vi "Convert_ERDs_JL.vi"(0 "New Header?":bool, 2 "ERD Name":string[](array[string]), 5 "ERD_Data_Bundled_Out":T1, 7 "Array":T11[](array[typedef]) {"ERD Number" format="%.0x"}, 11 "Error In":errorcluster) -> (6 "All_ERD_Data_Bundled_Brass":T1, 15 "Error Out":errorcluster)   [LabVIEW 2023]
doc: "This VI parses the data from ERDs in correct format, units, etc. It handles all hex to dec conversions, hex to enum, and hex to boolean conversions.\n\nIf Raw Data from ERD is blank string, then it will output values from shift register."
uses:
  Common/LabVIEW GEA2 Toolkit/GEA3/type defs/ERD Read Data Out.ctl
  type defs/All_Bundled_Data_JL.ctl
  Common/type defs/Version.ctl
  type defs/ERD_Always_Show_JL.ctl
  Common/type defs/CSV_File_String_Arrays.ctl
  Common/type defs/Fault Table Array.ctl
  Common/type defs/Fault_Table_Info.ctl
  type defs/Heat Control.ctl
  type defs/ERD_Commercial_Laundry.ctl
  Common/type defs/BootloaderVersion.ctl
  type defs/ERD_RJ45.ctl
panel:
  out "Numeric":i32
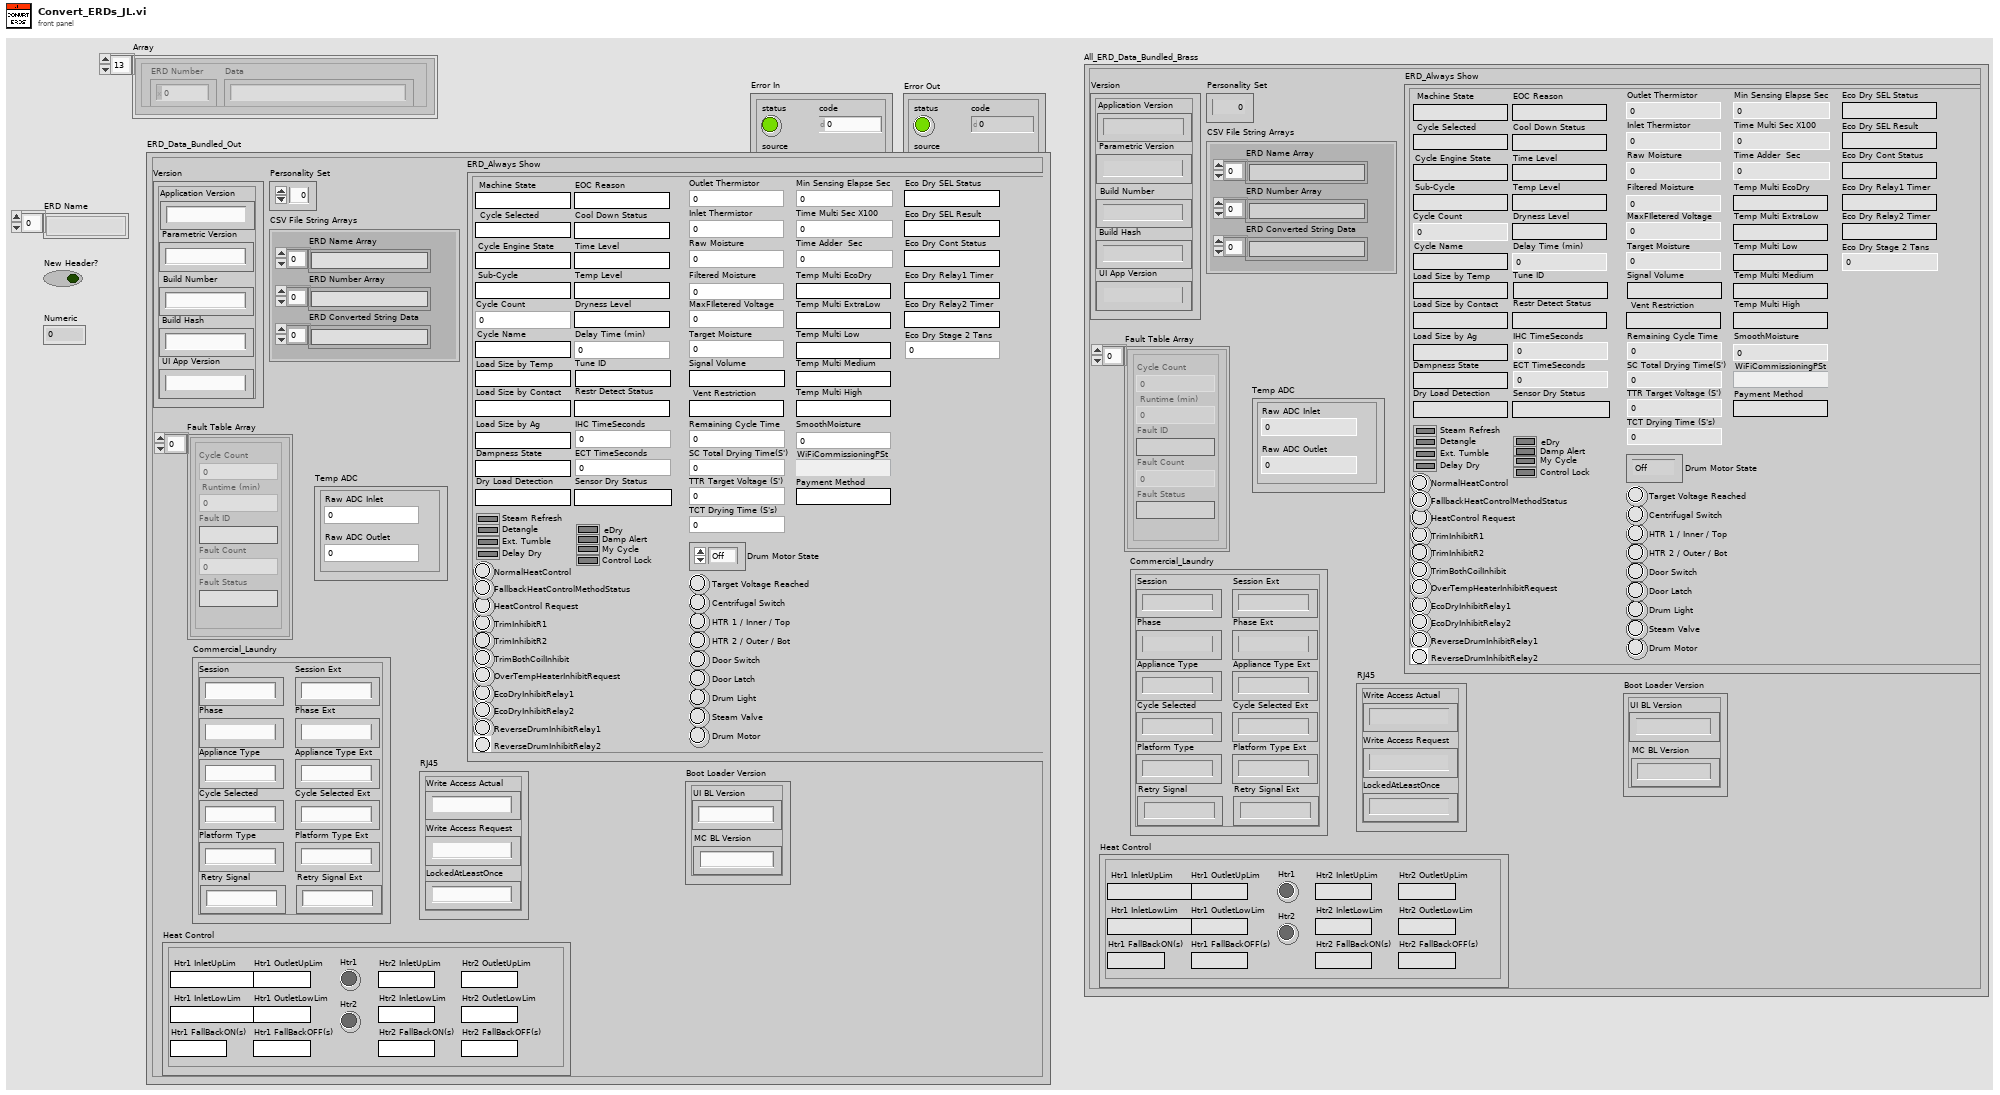
[diagram p1: front panel]
types:
  T1 = typedef "All_Bundled_Data_JL.ctl" = cluster{"Version":T2, "ERD_Always Show":T3, "Personality Set":u8, "CSV File String Arrays":T4, "Fault Table Array ":T5, "Heat Control":T7, "Temp ADC":cluster{"Raw ADC Outlet":u16, "Raw ADC Inlet":u16}, "Commercial_Laundry":T8, "Boot Loader Version":T9, "RJ45":T10}
  T2 = typedef "Version.ctl" = cluster{"Build Number":string, "Build Hash ":string, "Application Version":string, "Parametric Version":string, "UI App Version":string}
  T3 = typedef "ERD_Always_Show_JL.ctl" = cluster{"Inlet Thermistor":u16, "Machine State":string, "Filtered Moisture":u16, "Cycle Selected":string, "HTR 1 / Inner / Top":bool, "HTR 2 / Outer / Bot":bool, "Door Switch":bool, "Drum Light":bool, "Cycle Engine State":string, "Centrifugal Switch":bool, "Drum Motor":bool, "Cycle Count":u32, "Ext. Tumble":bool, "eDry":bool, "Temp Level":string, "Dryness Level":string, "Time Level":string, "Delay Time (min)":u16, "Steam Refresh":bool, "Damp Alert":bool, "Sub-Cycle":string, "Outlet Thermistor":u16, "Target Moisture":u16, "Remaining Cycle Time":u32, "Raw Moisture":u16, "Cycle Name":string, "My Cycle":bool, "Delay Dry":bool, "Detangle":bool, "Control Lock":bool, "Steam Valve":bool, "Door Latch":bool, "Signal Volume":string, "Tune ID":string, "Restr Detect Status":string, "Vent Restriction":string, "Load Size by Contact":string, "Load Size by Temp":string, "EOC Reason":string, "Sensor Dry Status":string, "Dampness State":string, "Target Voltage Reached":bool, "TrimInhibitR1":bool, "TrimInhibitR2":bool, "TrimBothCoilInhibit":bool, "NormalHeatControl":bool, "HeatControl Request":bool, "Cool Down Status":string, "EcoDryInhibitRelay1":bool, "EcoDryInhibitRelay2":bool, "ReverseDrumInhibitRelay1":bool, "ReverseDrumInhibitRelay2":bool, "OverTempHeaterInhibitRequest":bool, "FallbackHeatControlMethodStatus":bool, "IHC TimeSeconds":u32, "ECT TimeSeconds ":u32, "SC Total Drying Time(S')":u32, "TTR Target Voltage (S')":u32, "TCT Drying Time (S's)":u32, "Drum Motor State":enum16{"Off", "Cw", "Ccw", "Max"}, "Load Size by Ag":string, "MaxFIletered Voltage":u16, "Dry Load Detection":string, "Min Sensing Elapse Sec":u32, "Time Multi Sec X100":u32, "Time Adder  Sec":u32, "Temp Multi EcoDry":string, "Temp Multi ExtraLow":string, "Temp Multi Low ":string, "Temp Multi Medium":string, "Temp Multi High":string, "SmoothMoisture":u16, "Eco Dry SEL Status":string, "Eco Dry SEL Result":string, "Eco Dry Cont Status":string, "Eco Dry Relay1 Timer":string, "Eco Dry Relay2 Timer ":string, "Eco Dry Stage 2 Tans ":u32, "WiFiCommissioningPSt":string, "Payment Method":string}
  T4 = typedef "CSV_File_String_Arrays.ctl" = cluster{"ERD Number Array":string[], "ERD Name Array":string[], "ERD Converted String Data":string[]}
  T5 = typedef "Fault Table Array.ctl" = T6[]
  T6 = typedef "Fault_Table_Info.ctl" = cluster{"Cycle Count":u32, " Runtime (min) ":u32, "Fault Status":string, "Fault ID":string, "Fault Count":u16}
  T7 = typedef "Heat Control.ctl" = cluster{"Htr1 InletLowLim":string, "Htr1 InletUpLim":string, "Htr1 OutletLowLim":string, "Htr1 OutletUpLim":string, "Htr1 FallBackON(s)":string, "Htr1 FallBackOFF(s)":string, "Htr1":bool, "Htr2 InletLowLim":string, "Htr2 InletUpLim":string, "Htr2 OutletLowLim":string, "Htr2 OutletUpLim":string, "Htr2 FallBackON(s)":string, "Htr2 FallBackOFF(s)":string, "Htr2":bool}
  T8 = typedef "ERD_Commercial_Laundry.ctl" = cluster{"Session":string, "Phase":string, "Appliance Type":string, "Cycle Selected":string, "Platform Type":string, "Retry Signal":string, "Session Ext":string, "Phase Ext":string, "Appliance Type Ext":string, "Cycle Selected Ext":string, "Platform Type Ext":string, "Retry Signal Ext":string}
  T9 = typedef "BootloaderVersion.ctl" = cluster{"UI BL Version":string, "MC BL Version":string}
  T10 = typedef "ERD_RJ45.ctl" = cluster{"Write Access Actual":string, "Write Access Request":string, "LockedAtLeastOnce":string}
  T11 = typedef "ERD Read Data Out.ctl" = cluster{"ERD Number":u16, "Data":string}
  T12 = cluster{"Raw ADC Outlet":u16, "Raw ADC Inlet":u16}
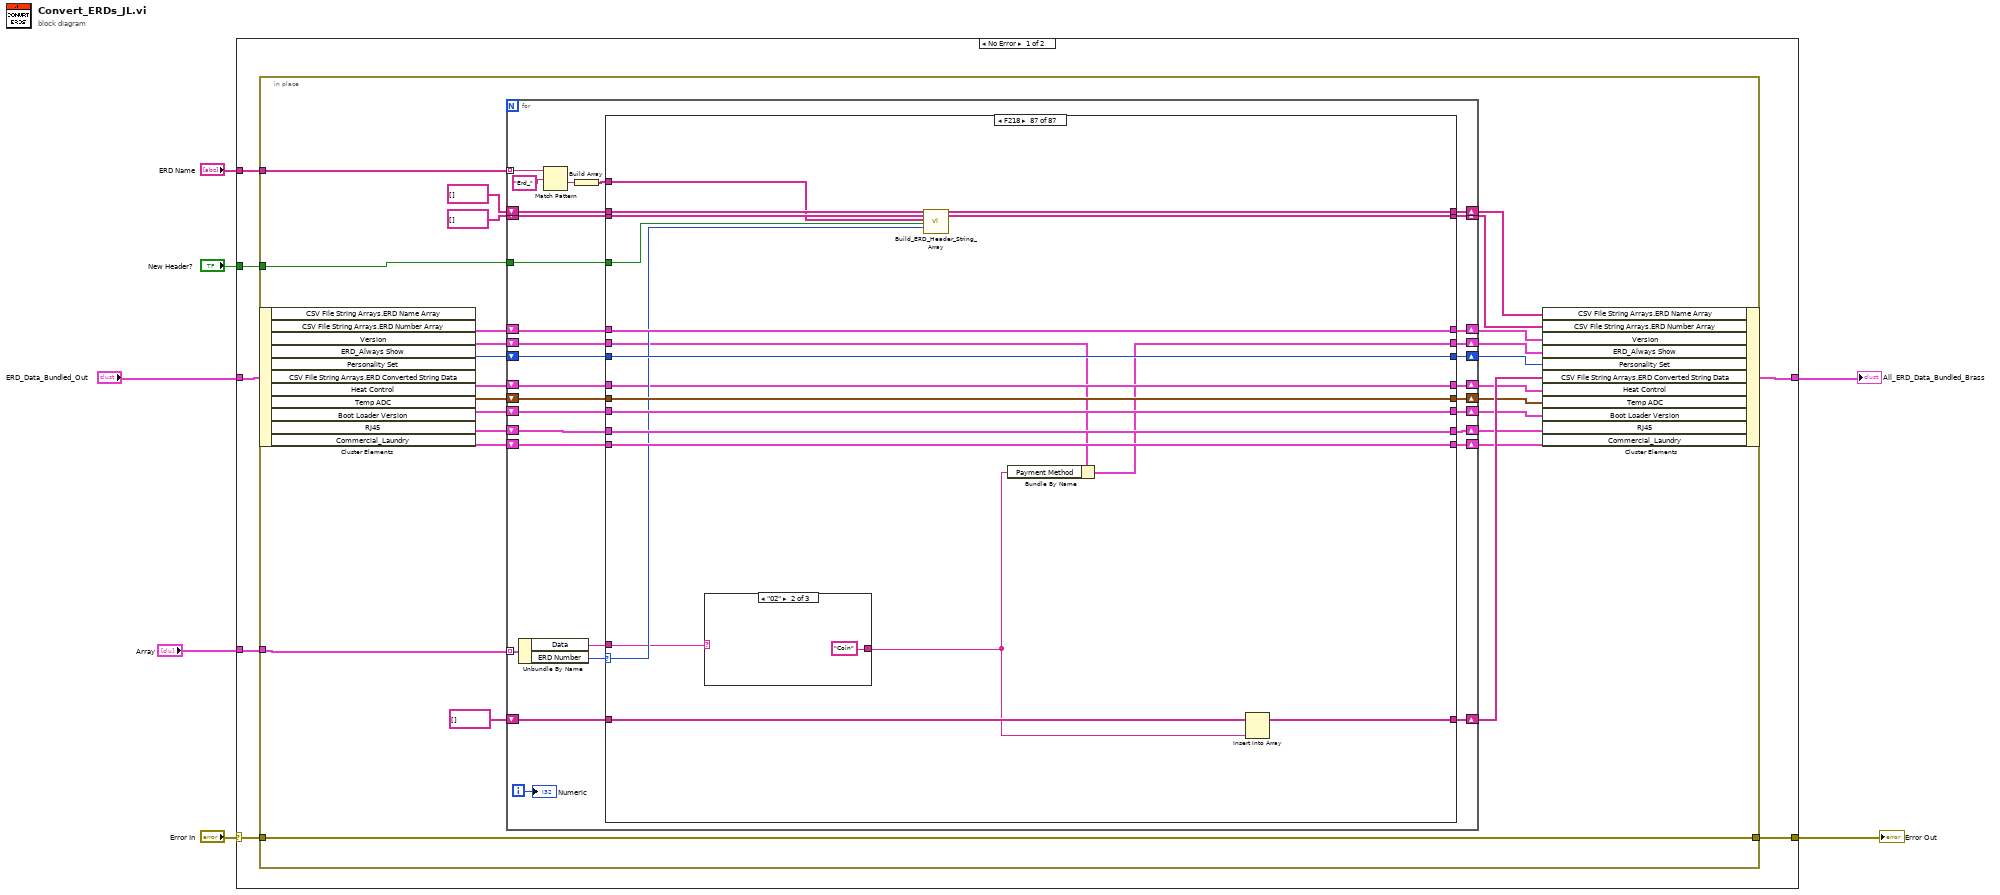
[diagram p0: block diagram]
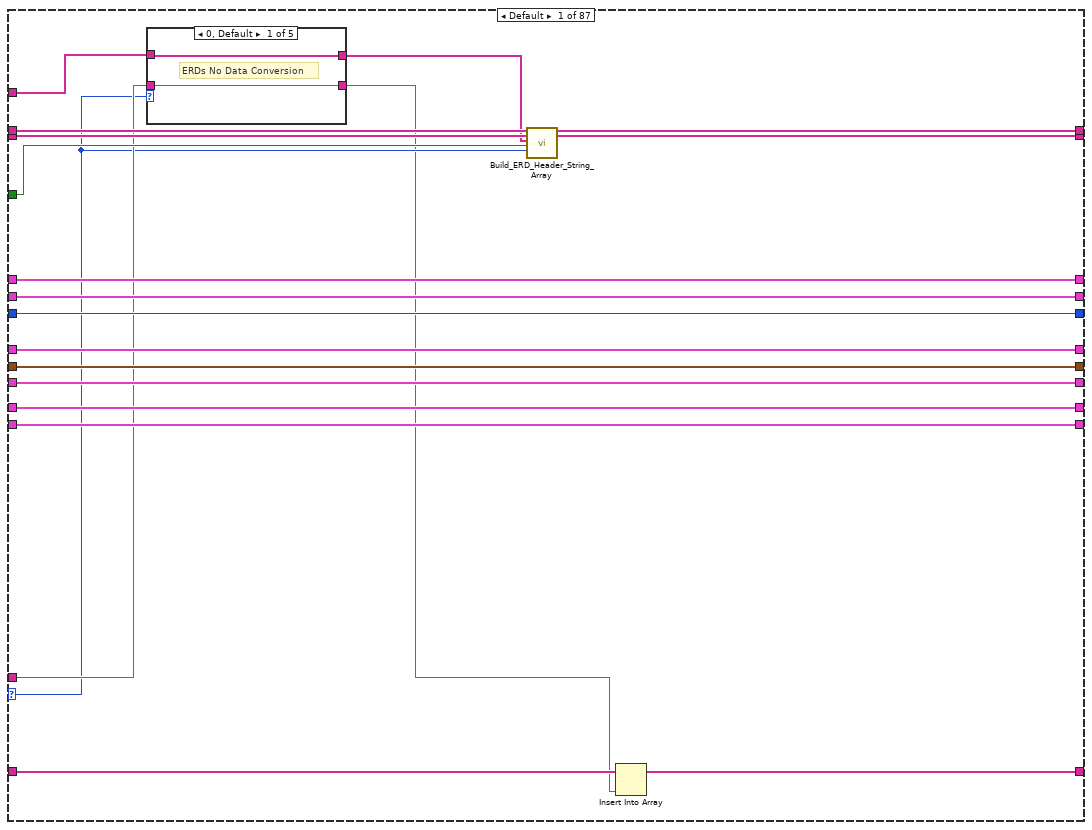
[diagram p2: hidden frame]
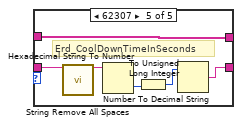
[diagram p6: hidden frame]
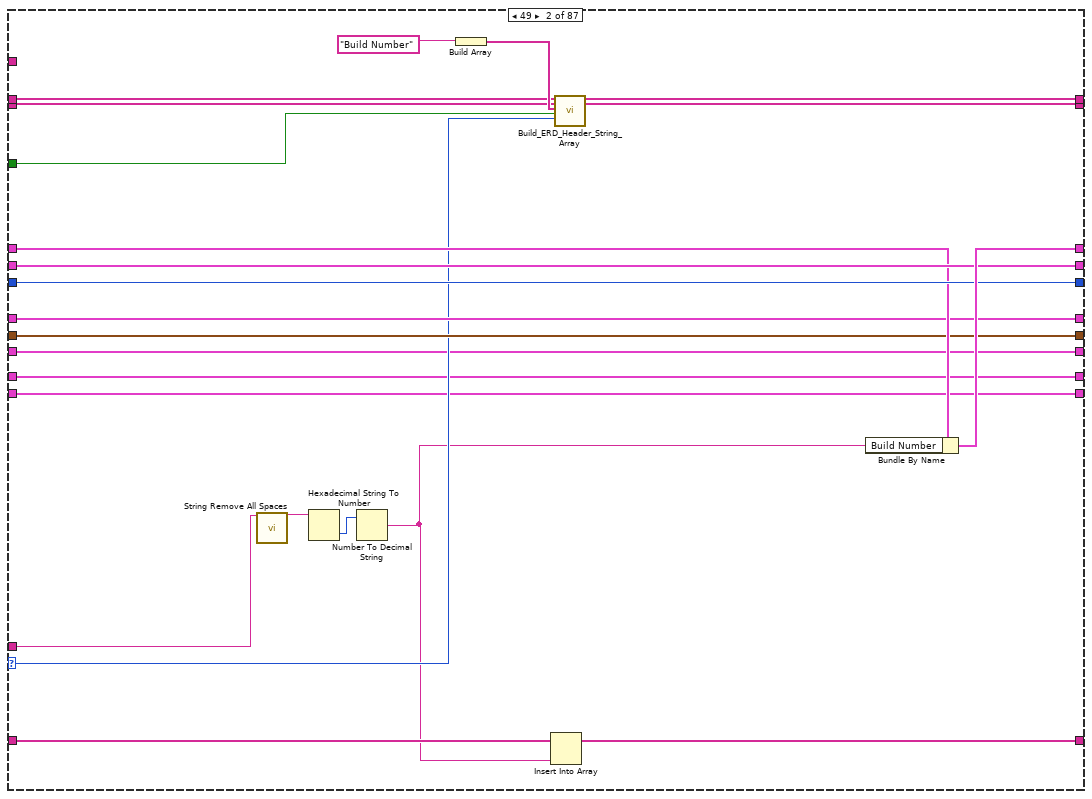
[diagram p7: hidden frame]
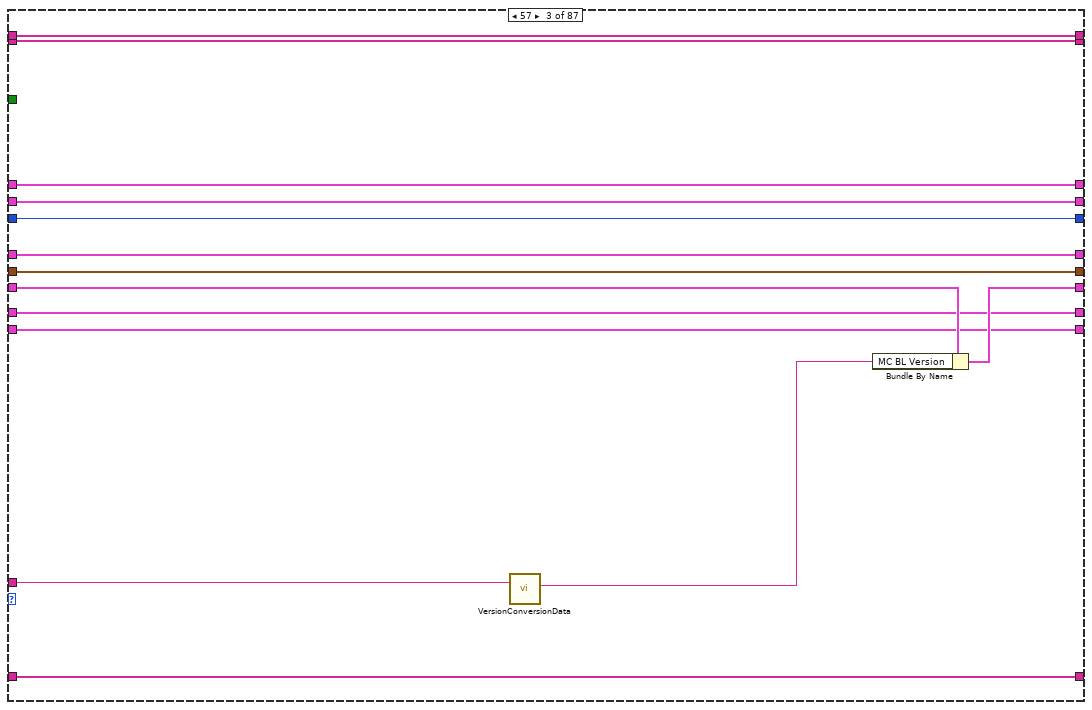
[diagram p8: hidden frame]
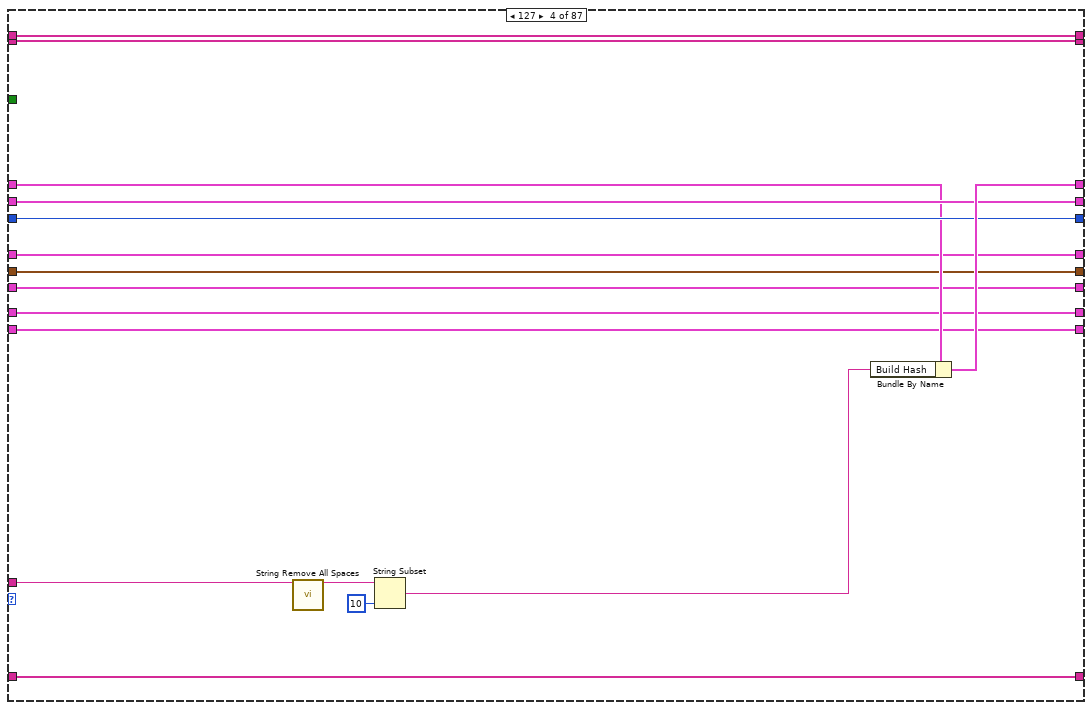
[diagram p9: hidden frame]
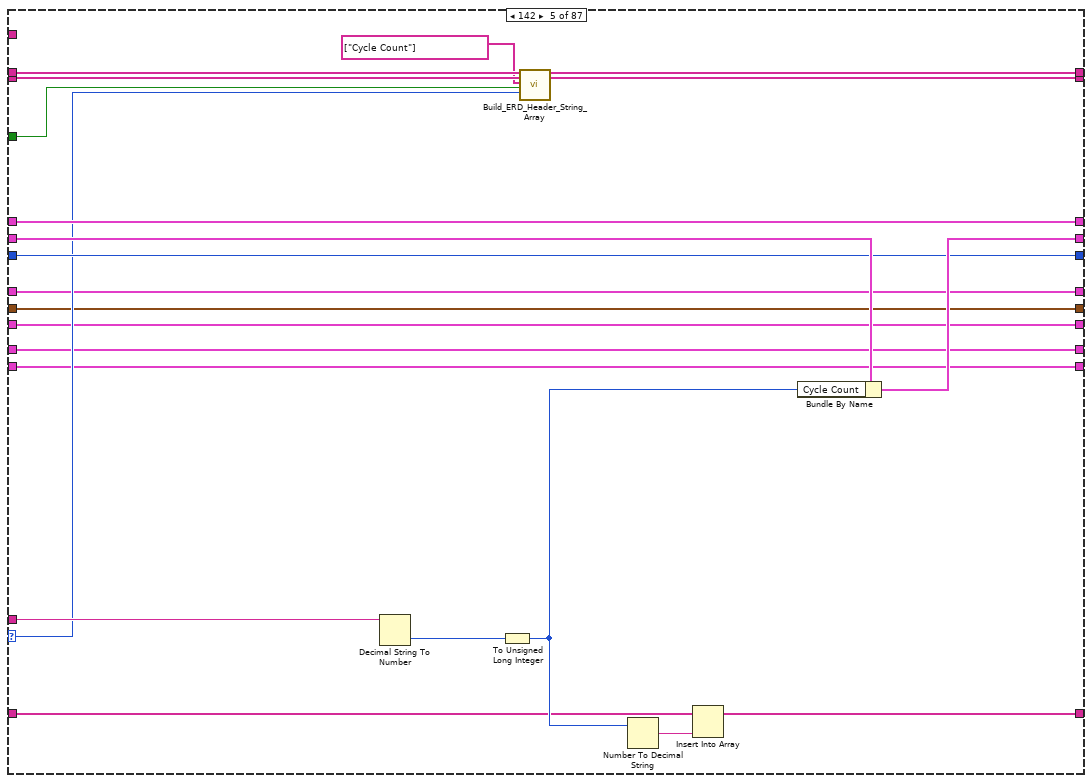
[diagram p10: hidden frame]
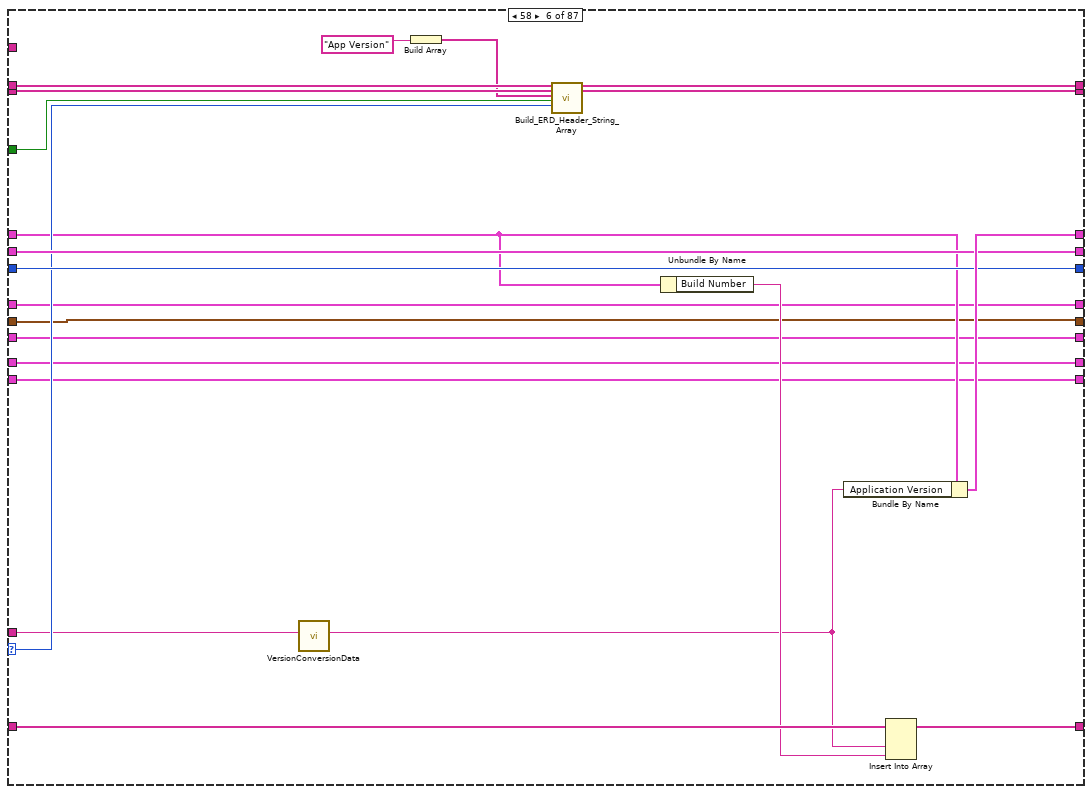
[diagram p11: hidden frame]
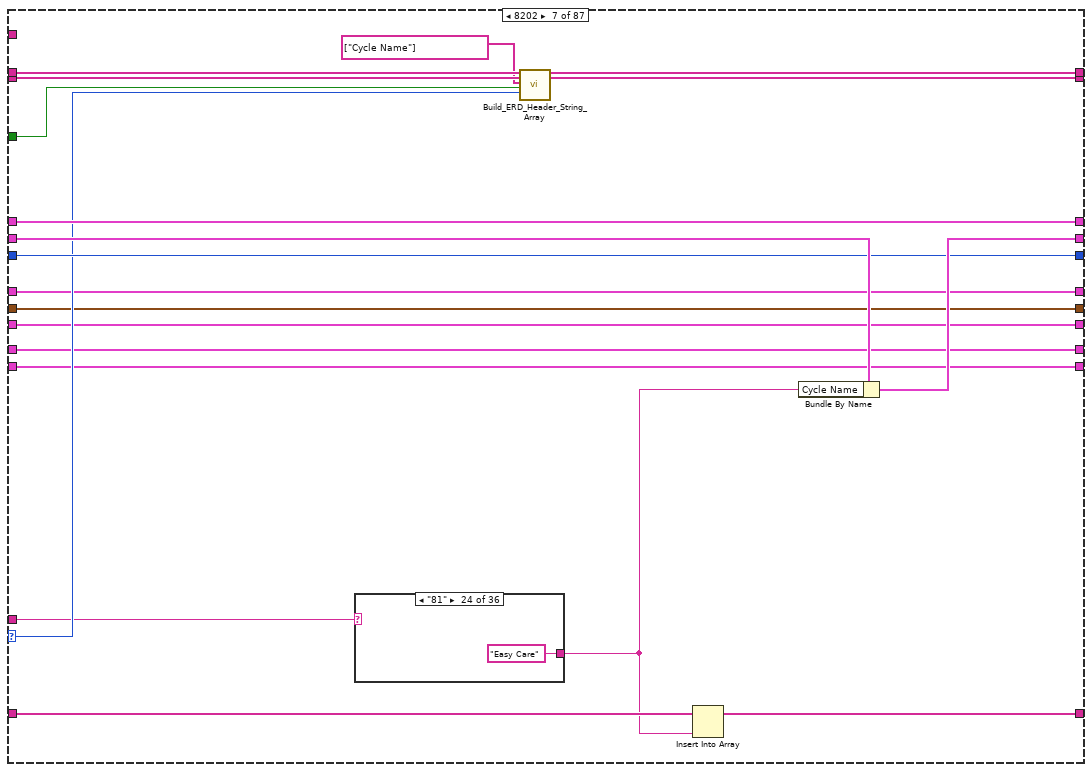
[diagram p12: hidden frame]
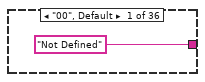
[diagram p13: hidden frame]
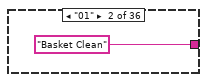
[diagram p14: hidden frame]
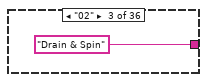
[diagram p15: hidden frame]
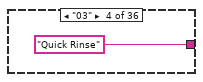
[diagram p16: hidden frame]
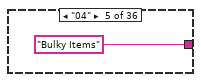
[diagram p17: hidden frame]
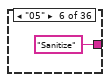
[diagram p18: hidden frame]
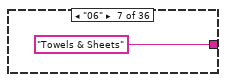
[diagram p19: hidden frame]
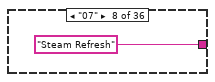
[diagram p20: hidden frame]
diagram:
  n1 = case shown="No Error" "Error In" {
    selector: "Error In" -> [w11 w2491]
    tunnel: "Array" -> [w14 _]
    tunnel: [w12 w2490] -> w5
    tunnel: "ERD_Data_Bundled_Out" -> [w13 w2489]
    tunnel: [w10 w2489] -> w4
    tunnel: "New Header?" -> [w9 _]
    tunnel: "ERD Name" -> [w8 _]
    frame No Error {
      n2 = in-place {
        in-place-border: w14 -> [w16]
        in-place-border: [w15] -> w12
        in-place-border: w11 -> [w15]
        in-place-border: w9 -> [w33]
        in-place-border: w8 -> [w21]
        n3 = in-place-cluster #1(w13) -> ("Version"=w39:T2, "ERD_Always Show"=w40:T3, "Personality Set"=w36:u8, "Heat Control"=w22:T7, "Temp ADC"=w25:T12, "Boot Loader Version"=w24:T9, "RJ45"=w19:T10, "Commercial_Laundry"=w17:T8)  [unwired: 3 out]
        n4 = for {
          shift-right: [w70] -> w37
          shift-left: w40 -> [w69]
          shift-right: [w67] -> w38
          shift-left: w39 -> [w68]
          shift-right: [w64] -> w35
          shift-left: w36 -> [w65]
          shift-right: [w62] -> w28
          shift-left: string[] [] ("ERD String Data") -> [w63]
          tunnel: w33 -> [w61]
          shift-right: [w57] -> w29
          shift-left: string[] [] ("ERD String Data") -> [w60]
          shift-right: [w58] -> w30
          shift-left: string[] [] ("ERD String Data") -> [w59]
          shift-right: [w50] -> w27
          shift-left: w22 -> [w56]
          shift-right: [w55] -> w26
          shift-left: w25 -> [w54]
          shift-right: [w51] -> w23
          shift-left: w24 -> [w52]
          tunnel: w21 -> [w49] mode=indexing
          shift-right: [w45] -> w20
          shift-left: w19 -> [w44]
          shift-right: [w43] -> w18
          shift-left: w17 -> [w42]
          tunnel: w16 -> [w41] mode=indexing
          i -> [w53]
          n5 = Unbundle By Name(w41) -> ("Data"=w71:string, "ERD Number"=w66:u16)
          n6 = Match Pattern(string=w49, regular expression="Erd_") -> (after substring=w46:string)  [unwired: 1 in, 3 out]
          n7 = Build Array(w46) -> (w47:string[])
          n8 = case shown="F218" w66 {
            selector: w66 -> [w73 w117 _ _ w169 w194 w212 w271 w296 w349 w380 w403 w431 w453 w498 w521 w544 w568 w587 w617 w649 w671 w694 w717 w740 w763 w787 w814 w836 w850 w877 w914 w933 w953 w982 w1005 w1036 w1063 w1086 w1111 w1135 w1158 w1181 w1203 w1226 w1272 w1290 w1313 w1336 w1359 w1382 w1405 w1428 w1451 w1471 w1499 w1554 w1612 w1642 w1673 w1693 w1722 w1747 w1770 w1793 w1816 w1842 w1872 w1897 w1920 w1937 w1965 w1988 w2011 w2037 w2061 w2081 w2102 w2143 w2170 w2188 w2212 w2239 w2266 w2313 w2406 w2478]
            tunnel: w71 -> [w74 w109 w130 w152 w180 w182 w209 w263 w289 w343 w393 w416 w427 w449 w468 w515 w538 w563 w595 w616 w648 w667 w691 w714 w737 w760 w782 w808 w828 w852 w883 w909 w930 w966 w981 w1016 w1046 w1077 w1100 w1121 w1149 w1172 w1195 w1216 w1239 w1267 w1301 w1324 w1347 w1370 w1393 w1416 w1439 w1462 w1485 w1492 w1564 w1622 w1652 w1684 w1704 w1732 w1758 w1781 w1804 w1827 w1853 w1865 w1889 w1912 w1947 w1964 w1987 w2010 w2048 w2053 w2092 w2112 w2141 w2167 w2182 w2205 w2233 w2260 w2282 w2375 w2469]
            tunnel: [w91 w127 w142 w157 w178 w201 w221 w279 w293 w358 w392 w415 w440 w462 w507 w530 w553 w576 w598 w629 w661 w685 w708 w731 w754 w777 w783 w804 w827 w859 w880 w907 w947 w965 w993 w1017 w1045 w1075 w1098 w1120 w1147 w1170 w1193 w1217 w1240 w1268 w1299 w1322 w1345 w1368 w1391 w1414 w1437 w1460 w1483 w1507 w1566 w1621 w1651 w1682 w1705 w1733 w1759 w1782 w1805 w1828 w1854 w1881 w1892 w1915 w1946 w1977 w2000 w2023 w2046 w2070 w2090 w2110 w2137 w2168 w2198 w2221 w2248 w2275 w2322 w2415 w2470] -> w70
            tunnel: w69 -> [w91 w127 w142 w157 w179 w201 w222 w279 w294 w359 w394 w417 w441 w463 w508 w531 w554 w577 w597 w630 w662 w682 w705 w728 w751 w774 w784 w805 w831 w858 w881 w908 w944 w967 w994 w1018 w1047 w1076 w1099 w1122 w1148 w1171 w1194 w1218 w1241 w1268 w1300 w1323 w1346 w1369 w1392 w1415 w1438 w1461 w1484 w1508 w1565 w1623 w1653 w1683 w1706 w1734 w1760 w1783 w1806 w1829 w1855 w1882 w1892 w1915 w1948 w1978 w2001 w2024 w2047 w2071 w2091 w2111 w2138 w2169 w2198 w2221 w2248 w2275 w2322 w2415 w2471]
            tunnel: w68 -> [w90 w125 w133 w153 w177 w193 w220 w278 w295 w357 w391 w414 w439 w461 w506 w529 w552 w575 w594 w628 w660 w684 w707 w730 w753 w776 w797 w806 w843 w870 w897 w924 w946 w964 w992 w1015 w1044 w1074 w1097 w1119 w1146 w1169 w1192 w1215 w1238 w1280 w1298 w1321 w1344 w1367 w1390 w1413 w1436 w1459 w1482 w1506 w1563 w1620 w1650 w1681 w1703 w1731 w1757 w1780 w1803 w1826 w1852 w1880 w1905 w1928 w1945 w1976 w1999 w2022 w2045 w2069 w2089 w2109 w2153 w2180 w2200 w2204 w2232 w2259 w2308 w2401 w2485]
            tunnel: [w90 w128 w133 w158 w177 w202 w220 w278 w295 w357 w391 w414 w439 w461 w506 w529 w552 w575 w594 w628 w660 w684 w707 w730 w753 w776 w797 w806 w843 w870 w897 w924 w946 w964 w992 w1015 w1044 w1074 w1097 w1119 w1146 w1169 w1192 w1215 w1238 w1280 w1298 w1321 w1344 w1367 w1390 w1413 w1436 w1459 w1482 w1506 w1563 w1620 w1650 w1681 w1703 w1731 w1757 w1780 w1803 w1826 w1852 w1880 w1905 w1928 w1945 w1976 w1999 w2022 w2045 w2069 w2089 w2109 w2153 w2180 w2199 w2204 w2232 w2259 w2308 w2401 w2485] -> w67
            tunnel: w65 -> [w89 w126 w141 w156 w176 w200 w219 _ w303 w356 w390 w413 w438 w460 w505 w528 w551 w574 w593 w627 w659 w681 w704 w727 w750 w773 w796 w821 w842 w869 w896 w923 w943 w963 w991 w1014 w1043 w1073 w1096 w1118 w1145 w1168 w1191 w1214 w1237 w1279 w1297 w1320 w1343 w1366 w1389 w1412 w1435 w1458 w1481 w1505 w1562 w1619 w1649 w1680 w1702 w1730 w1756 w1779 w1802 w1825 w1851 w1879 w1904 w1927 w1944 w1975 w1998 w2021 w2044 w2068 w2088 w2108 w2152 w2179 w2197 w2220 w2247 w2274 w2321 w2414 w2484]
            tunnel: [w89 w126 w141 w156 w176 w200 w219 w267 w303 w356 w390 w413 w438 w460 w505 w528 w551 w574 w593 w627 w659 w681 w704 w727 w750 w773 w796 w821 w842 w869 w896 w923 w943 w963 w991 w1014 w1043 w1073 w1096 w1118 w1145 w1168 w1191 w1214 w1237 w1279 w1297 w1320 w1343 w1366 w1389 w1412 w1435 w1458 w1481 w1505 w1562 w1619 w1649 w1680 w1702 w1730 w1756 w1779 w1802 w1825 w1851 w1879 w1904 w1927 w1944 w1975 w1998 w2021 w2044 w2068 w2088 w2108 w2152 w2179 w2197 w2220 w2247 w2274 w2321 w2414 w2484] -> w64
            tunnel: w63 -> [w85 w121 w138 w148 w174 w187 w217 w275 w300 w353 w384 w407 w435 w457 w502 w525 w548 w572 w591 w622 w653 w675 w698 w721 w744 w767 w791 w816 w834 w862 w887 w918 w937 w957 w987 w1011 w1040 w1067 w1090 w1115 w1139 w1162 w1185 w1208 w1231 w1276 w1294 w1317 w1340 w1363 w1386 w1409 w1432 w1455 w1475 w1503 w1558 w1616 w1646 w1677 w1699 w1728 w1753 w1776 w1799 w1822 w1848 w1876 w1901 w1924 w1941 w1969 w1992 w2015 w2041 w2065 w2085 w2106 w2148 w2174 w2192 w2216 w2243 w2270 w2317 w2410 w2474]
            tunnel: [w81 w120 w138 w148 w172 w196 w215 w273 w298 w351 w382 w405 w433 w455 w500 w523 w546 w570 w589 w620 w651 w673 w696 w719 w742 w765 w789 w812 w837 w865 w886 w916 w935 w955 w985 w1009 w1038 w1065 w1088 w1113 w1137 w1160 w1183 w1206 w1229 w1274 w1292 w1315 w1338 w1361 w1384 w1407 w1430 w1453 w1473 w1501 w1556 w1614 w1644 w1675 w1697 w1726 w1751 w1774 w1797 w1820 w1846 w1874 w1899 w1922 w1939 w1967 w1990 w2013 w2039 w2063 w2083 w2104 w2146 w2172 w2190 w2214 w2241 w2268 w2315 w2408 w2476] -> w62
            tunnel: w61 -> [w83 w115 _ _ w170 w195 w213 w272 w297 w350 w381 w404 w432 w454 w499 w522 w545 w569 w588 w619 w650 w672 w695 w718 w741 w764 w788 w815 w835 w861 w884 w915 w934 w954 w984 w1006 w1037 w1064 w1087 w1112 w1136 w1159 w1182 w1205 w1228 w1273 w1291 w1314 w1337 w1360 w1383 w1406 w1429 w1452 w1472 w1500 w1555 w1613 w1643 w1674 w1694 w1723 w1748 w1771 w1794 w1817 w1843 w1873 w1898 w1921 w1938 w1966 w1989 w2012 w2038 w2062 w2082 w2103 w2144 w2171 w2189 w2213 w2240 w2267 w2314 w2407 w2479]
            tunnel: w60 -> [w84 w119 w139 w154 w175 w188 w218 w276 w301 w354 w385 w408 w436 w458 w503 w526 w549 w573 w592 w623 w654 w676 w699 w722 w745 w768 w792 w817 w833 w863 w888 w919 w938 w958 w988 w1012 w1041 w1068 w1091 w1116 w1140 w1163 w1186 w1209 w1232 w1277 w1295 w1318 w1341 w1364 w1387 w1410 w1433 w1456 w1476 w1504 w1559 w1617 w1647 w1678 w1700 w1729 w1754 w1777 w1800 w1823 w1849 w1877 w1902 w1925 w1942 w1970 w1993 w2016 w2042 w2066 w2086 w2107 w2149 w2175 w2193 w2217 w2244 w2271 w2318 w2411 w2475]
            tunnel: w59 -> [w79 w113 w140 w155 w165 w199 w211 w269 w286 w346 w388 w411 w430 w452 w497 w520 w543 w567 w586 w625 w657 w679 w702 w725 w748 w771 w786 w810 w829 w856 w882 w911 w941 w962 w990 w1008 w1035 w1071 w1094 w1110 w1143 w1166 w1189 w1212 w1235 w1269 w1289 w1312 w1335 w1358 w1381 w1404 w1427 w1450 w1479 w1498 w1561 w1611 w1641 w1672 w1696 w1725 w1750 w1773 w1796 w1819 w1845 w1871 w1896 w1919 w1936 w1973 w1996 w2019 w2035 w2059 w2080 w2101 w2140 w2166 w2196 w2219 w2246 w2273 w2320 w2413 w2468]
            tunnel: [w80 w112 w140 w155 w164 w198 w210 w268 w285 w345 w387 w410 w429 w451 w496 w519 w542 w566 w585 w624 w656 w678 w701 w724 w747 w770 w785 w809 w830 w857 w878 w912 w940 w961 w989 w1007 w1034 w1070 w1093 w1109 w1142 w1165 w1188 w1211 w1234 w1271 w1288 w1311 w1334 w1357 w1380 w1403 w1426 w1449 w1478 w1497 w1560 w1610 w1640 w1671 w1695 w1724 w1749 w1772 w1795 w1818 w1844 w1870 w1895 w1918 w1935 w1972 w1995 w2018 w2034 w2058 w2079 w2100 w2135 w2165 w2195 w2218 w2245 w2272 w2319 w2412 w2467] -> w58
            tunnel: [w82 w118 w139 w154 w173 w197 w216 w274 w299 w352 w383 w406 w434 w456 w501 w524 w547 w571 w590 w621 w652 w674 w697 w720 w743 w766 w790 w813 w838 w864 w885 w917 w936 w956 w986 w1010 w1039 w1066 w1089 w1114 w1138 w1161 w1184 w1207 w1230 w1275 w1293 w1316 w1339 w1362 w1385 w1408 w1431 w1454 w1474 w1502 w1557 w1615 w1645 w1676 w1698 w1727 w1752 w1775 w1798 w1821 w1847 w1875 w1900 w1923 w1940 w1968 w1991 w2014 w2040 w2064 w2084 w2105 w2147 w2173 w2191 w2215 w2242 w2269 w2316 w2409 w2477] -> w57
            tunnel: w56 -> [w86 w124 w137 w147 w163 w191 w207 w266 w284 w339 w378 w401 w426 w448 w495 w517 w540 w564 w583 w614 w639 w669 w692 w715 w738 w761 w781 w811 w826 w855 w879 w913 w931 w952 w979 w1003 w1032 w1061 w1085 w1107 w1133 w1156 w1179 w1202 w1225 w1270 w1285 w1308 w1331 w1354 w1377 w1400 w1423 w1446 w1469 w1496 w1553 w1609 w1639 w1668 w1691 w1720 w1745 w1768 w1791 w1814 w1840 w1868 w1893 w1916 w1934 w1962 w1985 w2008 w2031 w2055 w2076 w2099 w2145 w2177 w2187 w2211 w2238 w2265 w2312 w2405 w2472]
            tunnel: [w86 w124 w137 w147 w163 w191 w207 w266 w284 w339 w378 w401 w426 w448 w495 w517 w540 w564 w583 w614 w639 w669 w692 w715 w738 w761 w781 w811 w826 w855 w879 w913 w931 w952 w979 w1003 w1032 w1061 w1085 w1107 w1133 w1156 w1179 w1202 w1225 w1264 w1285 w1308 w1331 w1354 w1377 w1400 w1423 w1446 w1469 w1496 w1553 w1609 w1639 w1668 w1691 w1720 w1745 w1768 w1791 w1814 w1840 w1868 w1893 w1916 w1934 w1962 w1985 w2008 w2031 w2055 w2076 w2099 w2145 w2177 w2187 w2211 w2238 w2265 w2312 w2405 w2472] -> w50
            tunnel: w54 -> [w88 w123 w136 w146 w162 w190 w206 w265 w283 w328 w377 w400 w425 w447 w494 w516 w539 w561 w582 w613 w638 w668 w689 w712 w735 w758 w795 w820 w841 w868 w895 w922 w928 w951 w978 w1002 w1031 w1060 w1084 w1106 w1132 w1155 w1178 w1201 w1224 w1261 w1284 w1307 w1330 w1353 w1376 w1399 w1422 w1445 w1468 w1495 w1552 w1607 w1637 w1667 w1690 w1719 w1744 w1767 w1790 w1813 w1839 w1867 w1891 w1914 w1932 w1961 w1984 w2007 w2030 w2054 w2075 w2098 w2151 w2178 w2186 w2210 w2237 w2264 w2311 w2404 w2483]
            tunnel: [w88 w123 w136 w146 w162 w190 w206 w265 w283 w328 w377 w400 w425 w447 w494 w516 w539 w561 w582 w613 w638 w668 w689 w712 w735 w758 w795 w820 w841 w868 w895 w922 w928 w951 w978 w1002 w1031 w1060 w1084 w1106 w1132 w1155 w1178 w1201 w1224 w1261 w1284 w1307 w1330 w1353 w1376 w1399 w1422 w1445 w1468 w1495 w1552 w1607 w1637 w1667 w1690 w1719 w1744 w1767 w1790 w1813 w1839 w1867 w1890 w1913 w1932 w1961 w1984 w2007 w2030 w2054 w2075 w2098 w2151 w2178 w2186 w2210 w2237 w2264 w2311 w2404 w2483] -> w55
            tunnel: w52 -> [w87 w114 w135 w145 w161 w189 w205 w264 w282 w327 w376 w399 w422 w444 w466 w511 w534 w558 w581 w612 w637 w665 w688 w711 w734 w757 w794 w819 w840 w867 w894 w921 w927 w950 w977 w1001 w1030 w1059 w1082 w1105 w1131 w1154 w1177 w1200 w1223 w1246 w1283 w1306 w1329 w1352 w1375 w1398 w1421 w1444 w1467 w1494 w1551 w1606 w1636 w1666 w1689 w1718 w1743 w1766 w1789 w1812 w1838 w1862 w1885 w1908 w1931 w1960 w1983 w2006 w2029 w2051 w2074 w2097 w2150 w2163 w2185 w2209 w2236 w2263 w2310 w2403 w2482]
            tunnel: [w87 w114 w134 w145 w161 w189 w205 w264 w282 w327 w376 w399 w422 w444 w466 w511 w534 w558 w581 w612 w637 w665 w688 w711 w734 w757 w794 w819 w840 w867 w894 w921 w927 w950 w977 w1001 w1030 w1059 w1082 w1105 w1131 w1154 w1177 w1200 w1223 w1246 w1283 w1306 w1329 w1352 w1375 w1398 w1421 w1444 w1467 w1494 w1551 w1606 w1636 w1666 w1689 w1718 w1743 w1766 w1789 w1812 w1838 w1862 w1885 w1908 w1931 w1960 w1983 w2006 w2029 w2051 w2074 w2097 w2150 w2163 w2185 w2209 w2236 w2263 w2310 w2403 w2482] -> w51
            tunnel: w47 -> [w77 _ _ _ _ _ _ w261 _ _ _ _ _ _ _ _ _ w557 w580 _ _ _ _ _ _ _ _ _ _ _ _ _ _ _ _ _ _ _ _ _ _ _ _ _ _ _ _ _ _ _ _ _ _ _ _ w1493 w1548 _ _ _ _ w1717 _ _ _ _ _ _ _ _ _ _ _ _ _ _ _ _ w2134 _ _ _ _ _ _ _ w2473]
            tunnel: [w76 w111 w132 w144 w160 w184 w204 w260 w281 w326 w375 w398 w421 w443 w465 w510 w533 w556 w579 w611 w636 w664 w687 w710 w733 w756 w780 w803 w825 w849 w876 w903 w926 w949 w976 w1000 w1029 w1058 w1081 w1104 w1130 w1153 w1176 w1199 w1222 w1245 w1282 w1305 w1328 w1351 w1374 w1397 w1420 w1443 w1466 w1489 w1547 w1605 w1635 w1665 w1688 w1716 w1742 w1765 w1788 w1811 w1837 w1861 w1884 w1907 w1930 w1959 w1982 w2005 w2028 w2050 w2073 w2096 w2133 w2162 w2184 w2202 w2230 w2257 w2306 w2399 w2481] -> w45
            tunnel: w44 -> [w76 w111 w132 w144 w160 w184 w204 w260 w281 w326 w375 w398 w421 w443 w465 w510 w533 w556 w579 w611 w636 w664 w687 w710 w733 w756 w780 w803 w825 w849 w876 w903 w926 w949 w976 w1000 w1029 w1058 w1081 w1104 w1130 w1153 w1176 w1199 w1222 w1245 w1282 w1305 w1328 w1351 w1374 w1397 w1420 w1443 w1466 w1489 w1547 w1605 w1635 w1665 w1688 w1716 w1742 w1765 w1788 w1811 w1837 w1861 w1884 w1907 w1930 w1959 w1982 w2005 w2028 w2050 w2073 w2096 w2133 w2162 w2184 w2203 w2231 w2258 w2306 w2399 w2481]
            tunnel: [w75 w110 w131 w143 w159 w183 w203 w259 w280 w325 w374 w397 w420 w442 w464 w509 w532 w555 w578 w610 w635 w663 w686 w709 w732 w755 w779 w802 w824 w848 w875 w902 w925 w948 w975 w999 w1028 w1057 w1080 w1103 w1129 w1152 w1175 w1198 w1221 w1244 w1281 w1304 w1327 w1350 w1373 w1396 w1419 w1442 w1465 w1488 w1546 w1604 w1634 w1664 w1687 w1715 w1741 w1764 w1787 w1810 w1836 w1860 w1883 w1906 w1929 w1958 w1981 w2004 w2027 w2049 w2072 w2095 w2132 w2161 w2183 w2208 w2235 w2262 w2281 w2374 w2480] -> w43
            tunnel: w42 -> [w75 w110 w131 w143 w159 w183 w203 w259 w280 w325 w374 w397 w420 w442 w464 w509 w532 w555 w578 w610 w635 w663 w686 w709 w732 w755 w779 w802 w824 w848 w875 w902 w925 w948 w975 w999 w1028 w1057 w1080 w1103 w1129 w1152 w1175 w1198 w1221 w1244 w1281 w1304 w1327 w1350 w1373 w1396 w1419 w1442 w1465 w1488 w1546 w1604 w1634 w1664 w1687 w1715 w1741 w1764 w1787 w1810 w1836 w1860 w1883 w1906 w1929 w1958 w1981 w2004 w2027 w2049 w2072 w2095 w2132 w2161 w2183 w2208 w2235 w2262 w2305 w2398 w2480]
            frame Default {
              n9 = case shown="0, Default" w73 {
                tunnel: [w92 w95 w97 w99 w105] -> w78
                tunnel: w77 -> [w92 w95 w97 w99 w105]
                tunnel: w74 -> [w93 w94 w96 w98 w102]
                tunnel: [w93 w94 w96 w98 w100] -> w72
                frame 0, Default {
                  # "ERDs No Data Conversion"
                }
                frame 65423 {
                  # "Consumer Error Mode"
                }
                frame 55 {
                  # "ServiceModeState"
                }
                frame 61811 {
                  # "WiFiCommissioningOption"
                }
                frame 62307 {
                  # "Erd_CoolDownTimeInSeconds"
                  n10 = call "String Remove All Spaces.vi"("Input String"=w102) -> ("Spaces Removed"=w103:string)  [unwired: 13 in, 1 out]
                  n11 = Hexadecimal String To Number(string=w103) -> (number=w104:u32)  [unwired: 2 in, 1 out]
                  n12 = To Unsigned Long Integer(number=w104) -> (unsigned 32bit integer=w101:u32)
                  n13 = Number To Decimal String(number=w101) -> (decimal integer string=w100:string)  [unwired: 1 in]
                }
              }
              n14 = call "Build_ERD_Header_String_Array.vi"("ERD Name Array In"=w84, "ERD Number Array In"=w85, "ERD Name List"=w78, "New Header?"=w83, "ERD Number"=w73) -> ("ERD Name Array Out"=w82:string[], "ERD Number Array Out"=w81:string[])  [unwired: 13 in]
              n15 = Insert Into Array(array=w79, new element=w72) -> (w80:string[])  [unwired: 1 in]
            }
            frame 49 {
              n16 = call "String Remove All Spaces.vi"("Input String"=w109) -> ("Spaces Removed"=w108:string)  [unwired: 13 in, 1 out]
              n17 = Hexadecimal String To Number(string=w108) -> (number=w106:u32)  [unwired: 2 in, 1 out]
              n18 = Number To Decimal String(number=w106) -> (decimal integer string=w107:string)  [unwired: 1 in]
              n19 = Build Array("Build Number") -> (w122:string[])
              n20 = Insert Into Array(array=w113, new element=w107) -> (w112:string[])  [unwired: 1 in]
              n21 = call "Build_ERD_Header_String_Array.vi"("ERD Name Array In"=w119, "ERD Number Array In"=w121, "ERD Name List"=w122, "New Header?"=w115, "ERD Number"=w117) -> ("ERD Name Array Out"=w118:string[], "ERD Number Array Out"=w120:string[])  [unwired: 13 in]
              n22 = Bundle By Name(cluster=w125, "Build Number"=w107) -> (w128:T2)
            }
            frame 57 {
              n23 = call "VersionConversionData.vi"("Version In"=w130) -> ("Version Out"=w129:string)  [unwired: 9 in, 1 out]
              n24 = Bundle By Name(cluster=w135, "MC BL Version"=w129) -> (w134:T9)
            }
            frame 127 {
              n25 = call "String Remove All Spaces.vi"("Input String"=w152) -> ("Spaces Removed"=w151:string)  [unwired: 13 in, 1 out]
              n26 = String Subset(string=w151, length (rest)=10 ("length (rest)")) -> (substring=w149:string)  [unwired: 1 in]
              n27 = Bundle By Name(cluster=w153, "Build Hash"=w149) -> (w158:T2)
            }
            frame 142 {
              n28 = Decimal String To Number(string=w180) -> (number=w167:i32)  [unwired: 2 in, 1 out]
              n29 = To Unsigned Long Integer(number=w167) -> (unsigned 32bit integer=w166:u32)
              n30 = call "Build_ERD_Header_String_Array.vi"("ERD Name Array In"=w175, "ERD Number Array In"=w174, "ERD Name List"=string[] ["Cycle Count"], "New Header?"=w170, "ERD Number"=w169) -> ("ERD Name Array Out"=w173:string[], "ERD Number Array Out"=w172:string[])  [unwired: 13 in]
              n31 = Number To Decimal String(number=w166) -> (decimal integer string=w168:string)  [unwired: 1 in]
              n32 = Insert Into Array(array=w165, new element=w168) -> (w164:string[])  [unwired: 1 in]
              n33 = Bundle By Name(cluster=w179, "Cycle Count"=w166) -> (w178:T3)
            }
            frame 58 {
              n34 = call "VersionConversionData.vi"("Version In"=w182) -> ("Version Out"=w181:string)  [unwired: 9 in, 1 out]
              n35 = Build Array("App Version" ("String")) -> (w185:string[])
              n36 = call "Build_ERD_Header_String_Array.vi"("ERD Name Array In"=w188, "ERD Number Array In"=w187, "ERD Name List"=w185, "New Header?"=w195, "ERD Number"=w194) -> ("ERD Name Array Out"=w197:string[], "ERD Number Array Out"=w196:string[])  [unwired: 13 in]
              n37 = Unbundle By Name(w193) -> ("Build Number"=w192:string)
              n38 = Bundle By Name(cluster=w193, "Application Version"=w181) -> (w202:T2)
              n39 = Insert Into Array(array=w199, new element #1=w181, new element #2=w192) -> (w198:string[])  [unwired: 1 in]
            }
            frame 8202 {
              n40 = case shown="\"81\"" w209 {
                tunnel: ["Not Defined" "Basket Clean" "Drain & Spin" "Quick Rinse" "Bulky Items" "Sanitize" "Towels & Sheets" "Steam Refresh" "Normal/Mixed" "Whites" "Dark Colors" "Jeans" "Hand Wash" "Delicates" "Speed Wash" "Heavy Duty" "Allergen" "Power Clean" "Rinse & Spin" "Single Item" "Colors" "Cold Wash" "Cottons" "Easy Care" "Active Wear" "Timed Dry" "Dewrinkle" "Air Fluff" "Steam Refresh" "Steam Dewrinkle" "Speed Dry" "Mixed" "Quick Dry" "Casuals" "Warm Up" "Energy Saver"] -> w208
                frame "00", Default {
                }
                frame "01" {
                }
                frame "02" {
                }
                frame "03" {
                }
                frame "04" {
                }
                frame "05" {
                }
                frame "06" {
                }
                frame "07" {
                }
                frame "08" {
                }
                frame "09" {
                }
                frame "0A" {
                }
                frame "0B" {
                }
                frame "0C" {
                }
                frame "0D" {
                }
                frame "0E" {
                }
                frame "0F" {
                }
                frame "10" {
                }
                frame "11" {
                }
                frame "12" {
                }
                frame "13" {
                }
                frame "14" {
                }
                frame "15" {
                }
                frame "80" {
                }
                frame "81" {
                }
                frame "82" {
                }
                frame "83" {
                }
                frame "84" {
                }
                frame "85" {
                }
                frame "86" {
                }
                frame "87" {
                }
                frame "88" {
                }
                frame "89" {
                }
                frame "8A" {
                }
                frame "8B" {
                }
                frame "8C" {
                }
                frame "8D" {
                }
              }
              n41 = call "Build_ERD_Header_String_Array.vi"("ERD Name Array In"=w218, "ERD Number Array In"=w217, "ERD Name List"=string[] ["Cycle Name"], "New Header?"=w213, "ERD Number"=w212) -> ("ERD Name Array Out"=w216:string[], "ERD Number Array Out"=w215:string[])  [unwired: 13 in]
              n42 = Insert Into Array(array=w211, new element=w208) -> (w210:string[])  [unwired: 1 in]
              n43 = Bundle By Name(cluster=w222, "Cycle Name"=w208) -> (w221:T3)
            }
            frame 65281 {
              n44 = call "String Remove All Spaces.vi"("Input String"=w263) -> ("Spaces Removed"=w262:string)  [unwired: 13 in, 1 out]
              n45 = Decimal String To Number(string=w262) -> (number=w277:i32)  [unwired: 2 in, 1 out]
              n46 = To Unsigned Byte Integer(number=w277) -> (unsigned 8bit integer=w267:u8)
              n47 = call "Build_ERD_Header_String_Array.vi"("ERD Name Array In"=w276, "ERD Number Array In"=w275, "ERD Name List"=w261, "New Header?"=w272, "ERD Number"=w271) -> ("ERD Name Array Out"=w274:string[], "ERD Number Array Out"=w273:string[])  [unwired: 13 in]
              n48 = Number To Decimal String(number=w267) -> (decimal integer string=w270:string)  [unwired: 1 in]
              n49 = Insert Into Array(array=w269, new element=w270) -> (w268:string[])  [unwired: 1 in]
            }
            frame 61443 {
              n50 = String Subset(string=w289, offset (0)=3, length (rest)=2 ("length (rest)")) -> (substring=w290:string)
              n51 = Hexadecimal String To Number(string=w290) -> (number=w288:u32)  [unwired: 2 in, 1 out]
              n52 = case shown="4" w288 {
                tunnel: ["Warning" ("Motor Profile") "Power Up" ("Motor Profile") "Power Down" ("Motor Profile") "Increase Sound" ("Motor Profile") "Decrease Sound" ("Motor Profile") "OK" ("Motor Profile") "OK Volume Key" ("Motor Profile") "Unavailable" ("Motor Profile") "Knob Turn" ("Motor Profile") "Notification 1" ("Motor Profile") "Notification 2" ("Motor Profile") "Notification 3" ("Motor Profile") "Notification Intro" ("Motor Profile") "Notification End" ("Motor Profile") "Feature ON" ("Motor Profile") "Feature OFF" ("Motor Profile") "Hold ON" ("Motor Profile") "Hold ON Volume" ("Motor Profile") "Hold OFF" ("Motor Profile") "Max" ("Motor Profile") "none" ("Motor Profile")] -> w287
                frame 0, Default {
                }
                frame 1 {
                }
                frame 2 {
                }
                frame 3 {
                }
                frame 4 {
                }
                frame 5 {
                }
                frame 6 {
                }
                frame 7 {
                }
                frame 8 {
                }
                frame 9 {
                }
                frame 10 {
                }
                frame 11 {
                }
                frame 12 {
                }
                frame 13 {
                }
                frame 14 {
                }
                frame 15 {
                }
                frame 16 {
                }
                frame 17 {
                }
                frame 18 {
                }
                frame 19 {
                }
                frame 20 {
                }
              }
              n53 = call "Build_ERD_Header_String_Array.vi"("ERD Name Array In"=w301, "ERD Number Array In"=w300, "ERD Name List"=string[] ["Tune ID"], "New Header?"=w297, "ERD Number"=w296) -> ("ERD Name Array Out"=w299:string[], "ERD Number Array Out"=w298:string[])  [unwired: 13 in]
              n54 = Insert Into Array(array=w286, new element=w287) -> (w285:string[])  [unwired: 1 in]
              n55 = Bundle By Name(cluster=w294, "Tune ID"=w287) -> (w293:T3)
            }
            frame 61457 {
              w337 = enum16{"Off", "Cw", "Ccw", "Max"}[] [enum."Off", enum."Cw", enum."Ccw", enum."Max"] items=["Off", "Cw", "Ccw", "Max"]
              n56 = for {
                N: 4 -> [_]
                tunnel: w343 -> [w369]
                tunnel: [w367] -> w331 mode=indexing
                tunnel: [w360] -> w338 mode=indexing
                i -> [w362]
                n57 = Increment(x=w362) -> (x+1=w361:i32)
                n58 = Multiply(x=w361, y=3) -> (x*y=w365:i32)
                n59 = Subtract(x=w365, y=3) -> (x-y=w363:i32)
                n60 = String Subset(string=w369, offset (0)=w363, length (rest)=2 ("length (rest)")) -> (substring=w360:string)
                n61 = call "HexStringToBoolean.vi"("Hex String"=w360) -> ("Boolean"=w367:bool)
              }
              n62 = Index Array(array=w338) -> (element=w336:string)  [unwired: 1 in]
              n63 = Decimal String To Number(string=w336) -> (number=w335:i32)  [unwired: 2 in, 1 out]
              n64 = Index Array(array=w337, index=w335) -> (element=w332:enum16{"Off", "Cw", "Ccw", "Max"})
              n65 = Greater Or Equal?(x=w335, y=1) -> (x >= y?=w330:bool)
              n66 = call "Build_ERD_Header_String_Array.vi"("ERD Name Array In"=w354, "ERD Number Array In"=w353, "ERD Name List"=string[] ["Drum Motor", "HTR 1 / Inner / Top", "HTR 2 / Outer / Bot", "Steam Valve"], "New Header?"=w350, "ERD Number"=w349) -> ("ERD Name Array Out"=w352:string[], "ERD Number Array Out"=w351:string[])  [unwired: 13 in]
              n67 = Insert Into Array(array=w331, new element=w330) -> (w329:bool[])  [unwired: 1 in]
              n68 = Index Array(array=w329) -> (element #1=w333:bool, element #2=w342:bool, element #3=w341:bool, element #4=w340:bool)  [unwired: 4 in]
              n69 = for {
                N: 4 -> [_]
                tunnel: [w371] -> w348 mode=indexing
                tunnel: w329 -> [w370] mode=indexing
                n70 = case shown="True" w370 {
                  tunnel: ["OFF" "ON"] -> w371
                  frame False {
                  }
                  frame True {
                  }
                }
              }
              n71 = Bundle By Name(cluster=w359, "Drum Motor State"=w332, "Drum Motor"=w333, "HTR 1 / Inner / Top"=w342, "HTR 2 / Outer / Bot"=w341, "Steam Valve"=w340) -> (w358:T3)
              n72 = Insert Into Array(array=w346, new element=w348) -> (w345:string[])  [unwired: 1 in]
            }
            frame 61459 {
              n73 = call "HexStringToBoolean.vi"("Hex String"=w393) -> ("Boolean"=w379:bool)
              n74 = case shown="False" w379 {
                tunnel: ["Open" "Closed"] -> w389
                frame False {
                }
                frame True {
                }
              }
              n75 = call "Build_ERD_Header_String_Array.vi"("ERD Name Array In"=w385, "ERD Number Array In"=w384, "ERD Name List"=string[] ["Door Switch"], "New Header?"=w381, "ERD Number"=w380) -> ("ERD Name Array Out"=w383:string[], "ERD Number Array Out"=w382:string[])  [unwired: 13 in]
              n76 = Insert Into Array(array=w388, new element=w389) -> (w387:string[])  [unwired: 1 in]
              n77 = Bundle By Name(cluster=w394, "Door Switch"=w379) -> (w392:T3)
            }
            frame 61460 {
              n78 = call "HexStringToBoolean.vi"("Hex String"=w416) -> ("Boolean"=w402:bool)
              n79 = case shown="True" w402 {
                tunnel: ["Unlatched" "Latched"] -> w412
                frame False {
                }
                frame True {
                }
              }
              n80 = call "Build_ERD_Header_String_Array.vi"("ERD Name Array In"=w408, "ERD Number Array In"=w407, "ERD Name List"=string[] ["Door Latch"], "New Header?"=w404, "ERD Number"=w403) -> ("ERD Name Array Out"=w406:string[], "ERD Number Array Out"=w405:string[])  [unwired: 13 in]
              n81 = Insert Into Array(array=w411, new element=w412) -> (w410:string[])  [unwired: 1 in]
              n82 = Bundle By Name(cluster=w417, "Door Latch"=w402) -> (w415:T3)
            }
            frame 61461 {
              n83 = Decimal String To Number(string=w427) -> (number=w423:i32)  [unwired: 2 in, 1 out]
              n84 = Number To Decimal String(number=w423) -> (decimal integer string=w424:string)  [unwired: 1 in]
              n85 = To Unsigned Word Integer(number=w423) -> (unsigned 16bit integer=w428:u16)
              n86 = call "Build_ERD_Header_String_Array.vi"("ERD Name Array In"=w436, "ERD Number Array In"=w435, "ERD Name List"=string[] ["Inlet Thermistor"], "New Header?"=w432, "ERD Number"=w431) -> ("ERD Name Array Out"=w434:string[], "ERD Number Array Out"=w433:string[])  [unwired: 13 in]
              n87 = Insert Into Array(array=w430, new element=w424) -> (w429:string[])  [unwired: 1 in]
              n88 = Bundle By Name(cluster=w441, "Inlet Thermistor"=w428) -> (w440:T3)
            }
            frame 61462 {
              n89 = Decimal String To Number(string=w449) -> (number=w446:i32)  [unwired: 2 in, 1 out]
              n90 = Number To Decimal String(number=w446) -> (decimal integer string=w445:string)  [unwired: 1 in]
              n91 = To Unsigned Word Integer(number=w446) -> (unsigned 16bit integer=w450:u16)
              n92 = call "Build_ERD_Header_String_Array.vi"("ERD Name Array In"=w458, "ERD Number Array In"=w457, "ERD Name List"=string[] ["Outlet Thermistor"], "New Header?"=w454, "ERD Number"=w453) -> ("ERD Name Array Out"=w456:string[], "ERD Number Array Out"=w455:string[])  [unwired: 13 in]
              n93 = Insert Into Array(array=w452, new element=w445) -> (w451:string[])  [unwired: 1 in]
              n94 = Bundle By Name(cluster=w463, "Outlet Thermistor"=w450) -> (w462:T3)
            }
            frame 63510 {
              n95 = call "String Remove All Spaces.vi"("Input String"=w468) -> ("Spaces Removed"=w467:string)  [unwired: 13 in, 1 out]
              n96 = String Subset(string=w467, offset (0)=0, length (rest)=4 ("offset (0)")) -> (substring=w491:string)
              n97 = String Subset(string=w467, offset (0)=4, length (rest)=4 ("offset (0)")) -> (substring=w490:string)
              n98 = String Subset(string=w467, offset (0)=8, length (rest)=4 ("offset (0)")) -> (substring=w485:string)
              n99 = String Subset(string=w467, offset (0)=12, length (rest)=4 ("offset (0)")) -> (substring=w479:string)
              n100 = String Subset(string=w467, offset (0)=16, length (rest)=4 ("offset (0)")) -> (substring=w480:string)
              n101 = Hexadecimal String To Number(string=w491) -> (number=w492:u32)  [unwired: 2 in, 1 out]
              n102 = Hexadecimal String To Number(string=w490) -> (number=w489:u32)  [unwired: 2 in, 1 out]
              n103 = Hexadecimal String To Number(string=w485) -> (number=w486:u32)  [unwired: 2 in, 1 out]
              n104 = Hexadecimal String To Number(string=w479) -> (number=w484:u32)  [unwired: 2 in, 1 out]
              n105 = Hexadecimal String To Number(string=w480) -> (number=w481:u32)  [unwired: 2 in, 1 out]
              n106 = Number To Decimal String(number=w492) -> (decimal integer string=w473:string)  [unwired: 1 in]
              n107 = Number To Decimal String(number=w489) -> (decimal integer string=w472:string)  [unwired: 1 in]
              n108 = Number To Decimal String(number=w486) -> (decimal integer string=w471:string)  [unwired: 1 in]
              n109 = Number To Decimal String(number=w484) -> (decimal integer string=w470:string)  [unwired: 1 in]
              n110 = Number To Decimal String(number=w481) -> (decimal integer string=w469:string)  [unwired: 1 in]
              n111 = call "Build_ERD_Header_String_Array.vi"("ERD Name Array In"=w503, "ERD Number Array In"=w502, "ERD Name List"=string[] ["Temp Multi EcoDry", "Temp Multi Extra Dry", "Temp Multi Low", "Temp Multi Medium", "Temp Multi High"], "New Header?"=w499, "ERD Number"=w498) -> ("ERD Name Array Out"=w501:string[], "ERD Number Array Out"=w500:string[])  [unwired: 13 in]
              n112 = Bundle By Name(cluster=w508, "Temp Multi EcoDry"=w473, "Temp Multi ExtraLow"=w472, "Temp Multi Low"=w471, "Temp Multi Medium"=w470, "Temp Multi High"=w469) -> (w507:T3)
              n113 = Insert Into Array(array=w497, new element #1=w473, new element #2=w472, new element #3=w471, new element #4=w470, new element #5=w469) -> (w496:string[])  [unwired: 1 in]
            }
            frame 61463 {
              n114 = call "String Remove All Spaces.vi"("Input String"=w515) -> ("Spaces Removed"=w514:string)  [unwired: 13 in, 1 out]
              n115 = Hexadecimal String To Number(string=w514) -> (number=w512:u32)  [unwired: 2 in, 1 out]
              n116 = To Unsigned Word Integer(number=w512) -> (unsigned 16bit integer=w518:u16)
              n117 = Number To Decimal String(number=w512) -> (decimal integer string=w513:string)  [unwired: 1 in]
              n118 = call "Build_ERD_Header_String_Array.vi"("ERD Name Array In"=w526, "ERD Number Array In"=w525, "ERD Name List"=string[] ["Filtered Moisture"], "New Header?"=w522, "ERD Number"=w521) -> ("ERD Name Array Out"=w524:string[], "ERD Number Array Out"=w523:string[])  [unwired: 13 in]
              n119 = Insert Into Array(array=w520, new element=w513) -> (w519:string[])  [unwired: 1 in]
              n120 = Bundle By Name(cluster=w531, "Filtered Moisture"=w518) -> (w530:T3)
            }
            frame 62242 {
              n121 = call "String Remove All Spaces.vi"("Input String"=w538) -> ("Spaces Removed"=w537:string)  [unwired: 13 in, 1 out]
              n122 = Hexadecimal String To Number(string=w537) -> (number=w535:u32)  [unwired: 2 in, 1 out]
              n123 = To Unsigned Word Integer(number=w535) -> (unsigned 16bit integer=w541:u16)
              n124 = Number To Decimal String(number=w535) -> (decimal integer string=w536:string)  [unwired: 1 in]
              n125 = call "Build_ERD_Header_String_Array.vi"("ERD Name Array In"=w549, "ERD Number Array In"=w548, "ERD Name List"=string[] ["SmoothMoistureReading"], "New Header?"=w545, "ERD Number"=w544) -> ("ERD Name Array Out"=w547:string[], "ERD Number Array Out"=w546:string[])  [unwired: 13 in]
              n126 = Insert Into Array(array=w543, new element=w536) -> (w542:string[])  [unwired: 1 in]
              n127 = Bundle By Name(cluster=w554, "SmoothMoisture"=w541) -> (w553:T3)
            }
            frame 61608 {
              n128 = call "String Remove All Spaces.vi"("Input String"=w563) -> ("Spaces Removed"=w562:string)  [unwired: 13 in, 1 out]
              n129 = Hexadecimal String To Number(string=w562) -> (number=w560:u32)  [unwired: 2 in, 1 out]
              n130 = Number To Decimal String(number=w560) -> (decimal integer string=w559:string)  [unwired: 1 in]
              n131 = To Unsigned Word Integer(number=w560) -> (unsigned 16bit integer=w565:u16)
              n132 = call "Build_ERD_Header_String_Array.vi"("ERD Name Array In"=w573, "ERD Number Array In"=w572, "ERD Name List"=w557, "New Header?"=w569, "ERD Number"=w568) -> ("ERD Name Array Out"=w571:string[], "ERD Number Array Out"=w570:string[])  [unwired: 13 in]
              n133 = Insert Into Array(array=w567, new element=w559) -> (w566:string[])  [unwired: 1 in]
              n134 = Bundle By Name(cluster=w577, "Target Moisture"=w565) -> (w576:T3)
            }
            frame 8192 {
              n135 = Decimal String To Number(string=w595) -> (number=w596:i32)  [unwired: 2 in, 1 out]
              n136 = case shown="5" w596 {
                tunnel: ["IDLE" "STANDBY" "RUN" "PAUSE" "EOC" "DSMDELAYRUN" "DELAY RUN" ("Profile Status") "DELAYPAUSE" ("Profile Status") "DRAIN TIME OUT" ("Profile Status") "COMMISIONING" ("Profile Status") "CLEANSPEAK" ("Profile Status")] -> w584
                frame 0, Default {
                }
                frame 1 {
                }
                frame 2 {
                }
                frame 3 {
                }
                frame 4 {
                }
                frame 5 {
                }
                frame 6 {
                }
                frame 7 {
                }
                frame 8 {
                }
                frame 9 {
                }
                frame 128 {
                }
              }
              n137 = call "Build_ERD_Header_String_Array.vi"("ERD Name Array In"=w592, "ERD Number Array In"=w591, "ERD Name List"=w580, "New Header?"=w588, "ERD Number"=w587) -> ("ERD Name Array Out"=w590:string[], "ERD Number Array Out"=w589:string[])  [unwired: 13 in]
              n138 = Insert Into Array(array=w586, new element=w584) -> (w585:string[])  [unwired: 1 in]
              n139 = Bundle By Name(cluster=w597, "Machine State"=w584) -> (w598:T3)
            }
            frame 8323 {
              n140 = case shown="\"02\"" w616 {
                tunnel: [FALSE TRUE] -> w615
                frame "01", Default {
                }
                frame "02" {
                }
              }
              n141 = case shown="True" w615 {
                tunnel: ["OFF" "ON"] -> w626
                frame False {
                }
                frame True {
                }
              }
              n142 = call "Build_ERD_Header_String_Array.vi"("ERD Name Array In"=w623, "ERD Number Array In"=w622, "ERD Name List"=string[] ["Control Lock"], "New Header?"=w619, "ERD Number"=w617) -> ("ERD Name Array Out"=w621:string[], "ERD Number Array Out"=w620:string[])  [unwired: 13 in]
              n143 = Insert Into Array(array=w625, new element=w626) -> (w624:string[])  [unwired: 1 in]
              n144 = Bundle By Name(cluster=w630, "Control Lock"=w615) -> (w629:T3)
            }
            frame 61478 {
              n145 = String Subset(string=w648, length (rest)=11 ("length (rest)")) -> (substring=w646:string)  [unwired: 1 in]
              n146 = call "String Remove All Spaces.vi"("Input String"=w646) -> ("Spaces Removed"=w645:string)  [unwired: 13 in, 1 out]
              n147 = Hexadecimal String To Number(string=w645) -> (number=w644:u32)  [unwired: 2 in, 1 out]
              n148 = To Double Precision Float(number=w644) -> (double precision float=w641:dbl)
              n149 = Divide(x=w641, y=60.0) -> (x/y=w643:dbl)
              n150 = call "Build_ERD_Header_String_Array.vi"("ERD Name Array In"=w654, "ERD Number Array In"=w653, "ERD Name List"=string[] ["Delay Time"], "New Header?"=w650, "ERD Number"=w649) -> ("ERD Name Array Out"=w652:string[], "ERD Number Array Out"=w651:string[])  [unwired: 13 in]
              n151 = To Unsigned Word Integer(number=w643) -> (unsigned 16bit integer=w642:u16)
              n152 = Number To Decimal String(number=w642) -> (decimal integer string=w658:string)  [unwired: 1 in]
              n153 = Bundle By Name(cluster=w662, "Delay Time (min)"=w642) -> (w661:T3)
              n154 = Insert Into Array(array=w657, new element=w658) -> (w656:string[])  [unwired: 1 in]
            }
            frame 61479 {
              n155 = call "String Remove All Spaces.vi"("Input String"=w667) -> ("Spaces Removed"=w666:string)  [unwired: 13 in, 1 out]
              n156 = Hexadecimal String To Number(string=w666) -> (number=w683:u32)  [unwired: 2 in, 1 out]
              n157 = To Unsigned Long Integer(number=w683) -> (unsigned 32bit integer=w670:u32)
              n158 = Bundle By Name(cluster=w682, "Remaining Cycle Time"=w670) -> (w685:T3)
              n159 = Number To Decimal String(number=w670) -> (decimal integer string=w680:string)  [unwired: 1 in]
              n160 = call "Build_ERD_Header_String_Array.vi"("ERD Name Array In"=w676, "ERD Number Array In"=w675, "ERD Name List"=string[] ["Remaing Cycle Time"], "New Header?"=w672, "ERD Number"=w671) -> ("ERD Name Array Out"=w674:string[], "ERD Number Array Out"=w673:string[])  [unwired: 13 in]
              n161 = Insert Into Array(array=w679, new element=w680) -> (w678:string[])  [unwired: 1 in]
            }
            frame 61698 {
              n162 = call "String Remove All Spaces.vi"("Input String"=w691) -> ("Spaces Removed"=w690:string)  [unwired: 13 in, 1 out]
              n163 = Hexadecimal String To Number(string=w690) -> (number=w706:u32)  [unwired: 2 in, 1 out]
              n164 = To Unsigned Long Integer(number=w706) -> (unsigned 32bit integer=w693:u32)
              n165 = Bundle By Name(cluster=w705, "IHC TimeSeconds"=w693) -> (w708:T3)
              n166 = Number To Decimal String(number=w693) -> (decimal integer string=w703:string)  [unwired: 1 in]
              n167 = call "Build_ERD_Header_String_Array.vi"("ERD Name Array In"=w699, "ERD Number Array In"=w698, "ERD Name List"=string[] ["Init HeatingTime Sec"], "New Header?"=w695, "ERD Number"=w694) -> ("ERD Name Array Out"=w697:string[], "ERD Number Array Out"=w696:string[])  [unwired: 13 in]
              n168 = Insert Into Array(array=w702, new element=w703) -> (w701:string[])  [unwired: 1 in]
            }
            frame 61606 {
              n169 = call "String Remove All Spaces.vi"("Input String"=w714) -> ("Spaces Removed"=w713:string)  [unwired: 13 in, 1 out]
              n170 = Hexadecimal String To Number(string=w713) -> (number=w729:u32)  [unwired: 2 in, 1 out]
              n171 = To Unsigned Long Integer(number=w729) -> (unsigned 32bit integer=w716:u32)
              n172 = Bundle By Name(cluster=w728, "ECT TimeSeconds"=w716) -> (w731:T3)
              n173 = Number To Decimal String(number=w716) -> (decimal integer string=w726:string)  [unwired: 1 in]
              n174 = call "Build_ERD_Header_String_Array.vi"("ERD Name Array In"=w722, "ERD Number Array In"=w721, "ERD Name List"=string[] ["Elapsed Cycle Time Sec"], "New Header?"=w718, "ERD Number"=w717) -> ("ERD Name Array Out"=w720:string[], "ERD Number Array Out"=w719:string[])  [unwired: 13 in]
              n175 = Insert Into Array(array=w725, new element=w726) -> (w724:string[])  [unwired: 1 in]
            }
            frame 61607 {
              n176 = call "String Remove All Spaces.vi"("Input String"=w737) -> ("Spaces Removed"=w736:string)  [unwired: 13 in, 1 out]
              n177 = Hexadecimal String To Number(string=w736) -> (number=w752:u32)  [unwired: 2 in, 1 out]
              n178 = To Unsigned Long Integer(number=w752) -> (unsigned 32bit integer=w739:u32)
              n179 = Bundle By Name(cluster=w751, "SC Total Drying Time(S')"=w739) -> (w754:T3)
              n180 = Number To Decimal String(number=w739) -> (decimal integer string=w749:string)  [unwired: 1 in]
              n181 = call "Build_ERD_Header_String_Array.vi"("ERD Name Array In"=w745, "ERD Number Array In"=w744, "ERD Name List"=string[] ["Sensing Ccle Total Drying Time sec"], "New Header?"=w741, "ERD Number"=w740) -> ("ERD Name Array Out"=w743:string[], "ERD Number Array Out"=w742:string[])  [unwired: 13 in]
              n182 = Insert Into Array(array=w748, new element=w749) -> (w747:string[])  [unwired: 1 in]
            }
            frame 61628 {
              n183 = call "String Remove All Spaces.vi"("Input String"=w760) -> ("Spaces Removed"=w759:string)  [unwired: 13 in, 1 out]
              n184 = Hexadecimal String To Number(string=w759) -> (number=w775:u32)  [unwired: 2 in, 1 out]
              n185 = To Unsigned Long Integer(number=w775) -> (unsigned 32bit integer=w762:u32)
              n186 = Bundle By Name(cluster=w774, "TTR Target Voltage (S')"=w762) -> (w777:T3)
              n187 = Number To Decimal String(number=w762) -> (decimal integer string=w772:string)  [unwired: 1 in]
              n188 = call "Build_ERD_Header_String_Array.vi"("ERD Name Array In"=w768, "ERD Number Array In"=w767, "ERD Name List"=string[] ["TTRTVoltage Seconds"], "New Header?"=w764, "ERD Number"=w763) -> ("ERD Name Array Out"=w766:string[], "ERD Number Array Out"=w765:string[])  [unwired: 13 in]
              n189 = Insert Into Array(array=w771, new element=w772) -> (w770:string[])  [unwired: 1 in]
            }
            frame 61728 {
              n190 = case shown="\"03\"" w782 {
                tunnel: ["Disabled" "Enabled" "Detect" "Finished"] -> w778
                frame "00", Default {
                }
                frame "01" {
                }
                frame "02" {
                }
                frame "03" {
                }
              }
              n191 = call "Build_ERD_Header_String_Array.vi"("ERD Name Array In"=w792, "ERD Number Array In"=w791, "ERD Name List"=string[] ["Eco Dry Sensor Dry Selector Status"], "New Header?"=w788, "ERD Number"=w787) -> ("ERD Name Array Out"=w790:string[], "ERD Number Array Out"=w789:string[])  [unwired: 13 in]
              n192 = Insert Into Array(array=w786, new element=w778) -> (w785:string[])  [unwired: 1 in]
              n193 = Bundle By Name(cluster=w784, "Eco Dry SEL Status"=w778) -> (w783:T3)
            }
            frame 61729 {
              n194 = case shown="\"00\", Default" w808 {
                tunnel: ["NormalDOD" "EDryDOD"] -> w807
                frame "00", Default {
                }
                frame "01" {
                }
              }
              n195 = call "Build_ERD_Header_String_Array.vi"("ERD Name Array In"=w817, "ERD Number Array In"=w816, "ERD Name List"=string[] ["Eco Dry Sensor Dry Selector Status"], "New Header?"=w815, "ERD Number"=w814) -> ("ERD Name Array Out"=w813:string[], "ERD Number Array Out"=w812:string[])  [unwired: 13 in]
              n196 = Insert Into Array(array=w810, new element=w807) -> (w809:string[])  [unwired: 1 in]
              n197 = Bundle By Name(cluster=w805, "Eco Dry SEL Result"=w807) -> (w804:T3)
            }
            frame 61736 {
              n198 = case shown="\"03\"" w828 {
                tunnel: ["Disabled" "Idle" "EcoDry Stage 1" "EcoDry Stage 2"] -> w832
                frame "00", Default {
                }
                frame "01" {
                }
                frame "02" {
                }
                frame "03" {
                }
              }
              n199 = call "Build_ERD_Header_String_Array.vi"("ERD Name Array In"=w833, "ERD Number Array In"=w834, "ERD Name List"=string[] ["Eco Dry Cont Status"], "New Header?"=w835, "ERD Number"=w836) -> ("ERD Name Array Out"=w838:string[], "ERD Number Array Out"=w837:string[])  [unwired: 13 in]
              n200 = Insert Into Array(array=w829, new element=w832) -> (w830:string[])  [unwired: 1 in]
              n201 = Bundle By Name(cluster=w831, "Eco Dry Cont Status"=w832) -> (w827:T3)
            }
            frame 61737 {
              n202 = String Subset(string=w852, offset (0)=12, length (rest)=2 ("length (rest)")) -> (substring=w851:string)
              n203 = case shown="\"03\"" w851 {
                tunnel: ["Disabled" "Not Inhibiting" "Active Inhibiting" "Max"] -> w860
                frame "00", Default {
                }
                frame "01" {
                }
                frame "02" {
                }
                frame "03" {
                }
              }
              n204 = call "Build_ERD_Header_String_Array.vi"("ERD Name Array In"=w863, "ERD Number Array In"=w862, "ERD Name List"=string[] ["Eco Dry Relay1 Timer"], "New Header?"=w861, "ERD Number"=w850) -> ("ERD Name Array Out"=w864:string[], "ERD Number Array Out"=w865:string[])  [unwired: 13 in]
              n205 = Bundle By Name(cluster=w858, "Eco Dry Relay1 Timer"=w860) -> (w859:T3)
              n206 = Insert Into Array(array=w856, new element=w860) -> (w857:string[])  [unwired: 1 in]
            }
            frame 61738 {
              n207 = String Subset(string=w883, offset (0)=12, length (rest)=2 ("length (rest)")) -> (substring=w889:string)
              n208 = case shown="\"03\"" w889 {
                tunnel: ["Disabled" "Not Inhibiting" "Active Inhibiting" "Max"] -> w892
                frame "00", Default {
                }
                frame "01" {
                }
                frame "02" {
                }
                frame "03" {
                }
              }
              n209 = call "Build_ERD_Header_String_Array.vi"("ERD Name Array In"=w888, "ERD Number Array In"=w887, "ERD Name List"=string[] ["Eco Dry Relay2 Timer"], "New Header?"=w884, "ERD Number"=w877) -> ("ERD Name Array Out"=w885:string[], "ERD Number Array Out"=w886:string[])  [unwired: 13 in]
              n210 = Bundle By Name(cluster=w881, "Eco Dry Relay2 Timer"=w892) -> (w880:T3)
              n211 = Insert Into Array(array=w882, new element=w892) -> (w878:string[])  [unwired: 1 in]
            }
            frame 61739 {
              n212 = call "String Remove All Spaces.vi"("Input String"=w909) -> ("Spaces Removed"=w905:string)  [unwired: 13 in, 1 out]
              n213 = Hexadecimal String To Number(string=w905) -> (number=w910:u32)  [unwired: 2 in, 1 out]
              n214 = To Unsigned Long Integer(number=w910) -> (unsigned 32bit integer=w904:u32)
              n215 = call "Build_ERD_Header_String_Array.vi"("ERD Name Array In"=w919, "ERD Number Array In"=w918, "ERD Name List"=string[] ["Eco Dry  Stage 2 Trans"], "New Header?"=w915, "ERD Number"=w914) -> ("ERD Name Array Out"=w917:string[], "ERD Number Array Out"=w916:string[])  [unwired: 13 in]
              n216 = Number To Decimal String(number=w904) -> (decimal integer string=w906:string)  [unwired: 1 in]
              n217 = Bundle By Name(cluster=w908, "Eco Dry Stage 2 Tans"=w904) -> (w907:T3)
              n218 = Insert Into Array(array=w911, new element=w906) -> (w912:string[])  [unwired: 1 in]
            }
            frame 61563 {
              n219 = call "String Remove All Spaces.vi"("Input String"=w930) -> ("Spaces Removed"=w929:string)  [unwired: 13 in, 1 out]
              n220 = Hexadecimal String To Number(string=w929) -> (number=w945:u32)  [unwired: 2 in, 1 out]
              n221 = To Unsigned Long Integer(number=w945) -> (unsigned 32bit integer=w932:u32)
              n222 = Bundle By Name(cluster=w944, "TCT Drying Time (S's)"=w932) -> (w947:T3)
              n223 = Number To Decimal String(number=w932) -> (decimal integer string=w942:string)  [unwired: 1 in]
              n224 = call "Build_ERD_Header_String_Array.vi"("ERD Name Array In"=w938, "ERD Number Array In"=w937, "ERD Name List"=string[] ["Timed Cycle Total Drying Time Seconds"], "New Header?"=w934, "ERD Number"=w933) -> ("ERD Name Array Out"=w936:string[], "ERD Number Array Out"=w935:string[])  [unwired: 13 in]
              n225 = Insert Into Array(array=w941, new element=w942) -> (w940:string[])  [unwired: 1 in]
            }
            frame 61480 {
              n226 = case shown="\"08\"" w966 {
                selector: w966 -> [w968 _ _ _ _ _ _]
                tunnel: [w968 "NONE" "FILL" "SOAK" "WASH" "RINSE" "SPIN"] -> w960
                frame Default {
                }
                frame "00" {
                }
                frame "01" {
                }
                frame "02" {
                }
                frame "04" {
                }
                frame "08" {
                }
                frame "10" {
                }
              }
              n227 = call "Build_ERD_Header_String_Array.vi"("ERD Name Array In"=w958, "ERD Number Array In"=w957, "ERD Name List"=string[] ["Sub-Cycle"], "New Header?"=w954, "ERD Number"=w953) -> ("ERD Name Array Out"=w956:string[], "ERD Number Array Out"=w955:string[])  [unwired: 13 in]
              n228 = Insert Into Array(array=w962, new element=w960) -> (w961:string[])  [unwired: 1 in]
              n229 = Bundle By Name(cluster=w967, "Sub-Cycle"=w960) -> (w965:T3)
            }
            frame 61483 {
              n230 = case shown="\"02\"" w981 {
                tunnel: ["Off" "High" "Medium" "Low"] -> w980
                frame "00", Default {
                }
                frame "01" {
                }
                frame "02" {
                }
                frame "04" {
                }
              }
              n231 = call "Build_ERD_Header_String_Array.vi"("ERD Name Array In"=w988, "ERD Number Array In"=w987, "ERD Name List"=string[] ["Signal Volume"], "New Header?"=w984, "ERD Number"=w982) -> ("ERD Name Array Out"=w986:string[], "ERD Number Array Out"=w985:string[])  [unwired: 13 in]
              n232 = Insert Into Array(array=w990, new element=w980) -> (w989:string[])  [unwired: 1 in]
              n233 = Bundle By Name(cluster=w994, "Signal Volume"=w980) -> (w993:T3)
            }
            frame 8272 {
              n234 = case shown="Default" w1016 {
                selector: w1016 -> [w1019 _ _ _ _ _ _ _ _]
                tunnel: [w1019 "Disabled" "No Heat" "Extra Low" "Low" "Medium" "High" "Max" "Don't Care"] -> w1004
                frame Default {
                }
                frame "00" {
                }
                frame "01" {
                }
                frame "02" {
                }
                frame "03" {
                }
                frame "04" {
                }
                frame "05" {
                }
                frame "06" {
                }
                frame "07" {
                }
              }
              n235 = call "Build_ERD_Header_String_Array.vi"("ERD Name Array In"=w1012, "ERD Number Array In"=w1011, "ERD Name List"=string[] ["Temp Level"], "New Header?"=w1006, "ERD Number"=w1005) -> ("ERD Name Array Out"=w1010:string[], "ERD Number Array Out"=w1009:string[])  [unwired: 13 in]
              n236 = Insert Into Array(array=w1008, new element=w1004) -> (w1007:string[])  [unwired: 1 in]
              n237 = Bundle By Name(cluster=w1018, "Temp Level"=w1004) -> (w1017:T3)
            }
            frame 8269 {
              n238 = case shown="\"255\"" w1046 {
                selector: w1046 -> [w1048 _ _ _ _ _ _ _ _]
                tunnel: [w1048 "Disabled" "Damp" "Less Dry" "Dry" "More Dry" "Extra Dry" "Max" "Don't Care"] -> w1033
                frame Default {
                }
                frame "00" {
                }
                frame "01" {
                }
                frame "02" {
                }
                frame "03" {
                }
                frame "04" {
                }
                frame "05" {
                }
                frame "06" {
                }
                frame "255" {
                }
              }
              n239 = call "Build_ERD_Header_String_Array.vi"("ERD Name Array In"=w1041, "ERD Number Array In"=w1040, "ERD Name List"=string[] ["Dryness Level"], "New Header?"=w1037, "ERD Number"=w1036) -> ("ERD Name Array Out"=w1039:string[], "ERD Number Array Out"=w1038:string[])  [unwired: 13 in]
              n240 = Insert Into Array(array=w1035, new element=w1033) -> (w1034:string[])  [unwired: 1 in]
              n241 = Bundle By Name(cluster=w1047, "Dryness Level"=w1033) -> (w1045:T3)
            }
            frame 8262 {
              n242 = call "HexStringToBoolean.vi"("Hex String"=w1077) -> ("Boolean"=w1062:bool)
              n243 = case shown="True" w1062 {
                tunnel: ["OFF" "ON"] -> w1072
                frame False {
                }
                frame True {
                }
              }
              n244 = Insert Into Array(array=w1071, new element=w1072) -> (w1070:string[])  [unwired: 1 in]
              n245 = call "Build_ERD_Header_String_Array.vi"("ERD Name Array In"=w1068, "ERD Number Array In"=w1067, "ERD Name List"=string[] ["eDry"], "New Header?"=w1064, "ERD Number"=w1063) -> ("ERD Name Array Out"=w1066:string[], "ERD Number Array Out"=w1065:string[])  [unwired: 13 in]
              n246 = Bundle By Name(cluster=w1076, "eDry"=w1062) -> (w1075:T3)
            }
            frame 61600 {
              n247 = call "HexStringToBoolean.vi"("Hex String"=w1100) -> ("Boolean"=w1083:bool)
              n248 = case shown="False" w1083 {
                tunnel: ["OFF" "ON"] -> w1095
                frame False {
                }
                frame True {
                }
              }
              n249 = Insert Into Array(array=w1094, new element=w1095) -> (w1093:string[])  [unwired: 1 in]
              n250 = call "Build_ERD_Header_String_Array.vi"("ERD Name Array In"=w1091, "ERD Number Array In"=w1090, "ERD Name List"=string[] ["HeatControlRequest"], "New Header?"=w1087, "ERD Number"=w1086) -> ("ERD Name Array Out"=w1089:string[], "ERD Number Array Out"=w1088:string[])  [unwired: 13 in]
              n251 = Bundle By Name(cluster=w1099, "HeatControl Request"=w1083) -> (w1098:T3)
            }
            frame 8311 {
              n252 = case shown="\"05\"" w1121 {
                tunnel: ["TimeLevelOption_5" "TimeLevelOption_Disabled" "TimeLevelOption_1" "TimeLevelOption_2" "TimeLevelOption_3" "TimeLevelOption_4"] -> w1108
                frame "05" {
                }
                frame "00", Default {
                }
                frame "01" {
                }
                frame "02" {
                }
                frame "03" {
                }
                frame "04" {
                }
              }
              n253 = call "Build_ERD_Header_String_Array.vi"("ERD Name Array In"=w1116, "ERD Number Array In"=w1115, "ERD Name List"=string[] ["Time Level"], "New Header?"=w1112, "ERD Number"=w1111) -> ("ERD Name Array Out"=w1114:string[], "ERD Number Array Out"=w1113:string[])  [unwired: 13 in]
              n254 = Insert Into Array(array=w1110, new element=w1108) -> (w1109:string[])  [unwired: 1 in]
              n255 = Bundle By Name(cluster=w1122, "Time Level"=w1108) -> (w1120:T3)
            }
            frame 8275 {
              n256 = call "HexStringToBoolean.vi"("Hex String"=w1149) -> ("Boolean"=w1134:bool)
              n257 = case shown="True" w1134 {
                tunnel: ["OFF" "ON"] -> w1144
                frame False {
                }
                frame True {
                }
              }
              n258 = Insert Into Array(array=w1143, new element=w1144) -> (w1142:string[])  [unwired: 1 in]
              n259 = call "Build_ERD_Header_String_Array.vi"("ERD Name Array In"=w1140, "ERD Number Array In"=w1139, "ERD Name List"=string[] ["Extended Tumble"], "New Header?"=w1136, "ERD Number"=w1135) -> ("ERD Name Array Out"=w1138:string[], "ERD Number Array Out"=w1137:string[])  [unwired: 13 in]
              n260 = Bundle By Name(cluster=w1148, "Ext. Tumble"=w1134) -> (w1147:T3)
            }
            frame 8266 {
              n261 = call "HexStringToBoolean.vi"("Hex String"=w1172) -> ("Boolean"=w1157:bool)
              n262 = case shown="True" w1157 {
                tunnel: ["OFF" "ON"] -> w1167
                frame False {
                }
                frame True {
                }
              }
              n263 = Insert Into Array(array=w1166, new element=w1167) -> (w1165:string[])  [unwired: 1 in]
              n264 = call "Build_ERD_Header_String_Array.vi"("ERD Name Array In"=w1163, "ERD Number Array In"=w1162, "ERD Name List"=string[] ["Damp Alert"], "New Header?"=w1159, "ERD Number"=w1158) -> ("ERD Name Array Out"=w1161:string[], "ERD Number Array Out"=w1160:string[])  [unwired: 13 in]
              n265 = Bundle By Name(cluster=w1171, "Damp Alert"=w1157) -> (w1170:T3)
            }
            frame 61501 {
              n266 = call "HexStringToBoolean.vi"("Hex String"=w1195) -> ("Boolean"=w1180:bool)
              n267 = case shown="True" w1180 {
                tunnel: ["OFF" "ON"] -> w1190
                frame False {
                }
                frame True {
                }
              }
              n268 = Insert Into Array(array=w1189, new element=w1190) -> (w1188:string[])  [unwired: 1 in]
              n269 = call "Build_ERD_Header_String_Array.vi"("ERD Name Array In"=w1186, "ERD Number Array In"=w1185, "ERD Name List"=string[] ["Detangle"], "New Header?"=w1182, "ERD Number"=w1181) -> ("ERD Name Array Out"=w1184:string[], "ERD Number Array Out"=w1183:string[])  [unwired: 13 in]
              n270 = Bundle By Name(cluster=w1194, "Detangle"=w1180) -> (w1193:T3)
            }
            frame 61503 {
              n271 = call "HexStringToBoolean.vi"("Hex String"=w1216) -> ("Boolean"=w1210:bool)
              n272 = case shown="True" w1210 {
                tunnel: ["OFF" "ON"] -> w1213
                frame False {
                }
                frame True {
                }
              }
              n273 = call "Build_ERD_Header_String_Array.vi"("ERD Name Array In"=w1209, "ERD Number Array In"=w1208, "ERD Name List"=string[] ["Delay Dry"], "New Header?"=w1205, "ERD Number"=w1203) -> ("ERD Name Array Out"=w1207:string[], "ERD Number Array Out"=w1206:string[])  [unwired: 13 in]
              n274 = Insert Into Array(array=w1212, new element=w1213) -> (w1211:string[])  [unwired: 1 in]
              n275 = Bundle By Name(cluster=w1218, "Delay Dry"=w1210) -> (w1217:T3)
            }
            frame 61510 {
              n276 = call "HexStringToBoolean.vi"("Hex String"=w1239) -> ("Boolean"=w1233:bool)
              n277 = case shown="True" w1233 {
                tunnel: ["OFF" "ON"] -> w1236
                frame False {
                }
                frame True {
                }
              }
              n278 = call "Build_ERD_Header_String_Array.vi"("ERD Name Array In"=w1232, "ERD Number Array In"=w1231, "ERD Name List"=string[] ["My Cycle"], "New Header?"=w1228, "ERD Number"=w1226) -> ("ERD Name Array Out"=w1230:string[], "ERD Number Array Out"=w1229:string[])  [unwired: 13 in]
              n279 = Insert Into Array(array=w1235, new element=w1236) -> (w1234:string[])  [unwired: 1 in]
              n280 = Bundle By Name(cluster=w1241, "My Cycle"=w1233) -> (w1240:T3)
            }
            frame 61549 {
              n281 = call "Heat Control Parse (SubVI).vi"("Data"=w1267, "Heat Control in"=w1270) -> ("Heat Control out"=w1264:T7)  [unwired: 9 in]
              n282 = Unbundle By Name(w1264) -> ("Htr1 InletLowLim"=w1260:string, "Htr1 InletUpLim"=w1259:string, "Htr1 OutletLowLim"=w1258:string, "Htr1 OutletUpLim"=w1257:string, "Htr1 FallBackON(s)"=w1256:string, "Htr1 FallBackOFF(s)"=w1255:string, "Htr1"=w1263:bool, "Htr2 InletLowLim"=w1253:string, "Htr2 InletUpLim"=w1252:string, "Htr2 OutletLowLim"=w1251:string, "Htr2 OutletUpLim"=w1250:string, "Htr2 FallBackON(s)"=w1249:string, "Htr2 FallBackOFF(s)"=w1248:string, "Htr2"=w1262:bool)
              n283 = Boolean To (0,1)(Boolean=w1262) -> (0, 1=w1265:i16)
              n284 = Number To Decimal String(number=w1265) -> (decimal integer string=w1247:string)  [unwired: 1 in]
              n285 = call "Build_ERD_Header_String_Array.vi"("ERD Name Array In"=w1277, "ERD Number Array In"=w1276, "ERD Name List"=string[] ["Htr1 Inlet Low Limit", "Htr 1 Upper Temp Limit", "Htr 1 Lower Limit Outlet ", "Htr 1 Upper Limit Outlet ", "Htr 1 Fallback On Time in Sec", "Htr 1 Fallback Off Time in Sec", "Htr 1 Relay Enable Status", "Htr2 Inlet Low Limit", "Htr 2 Upper Temp Limit", "Htr 2 Upper Limit Outlet ", "Htr2 Upper Limit Outlet ", "Htr 2 Fallback On Time in Sec", "Htr 2 Fallback Off Time in Sec", "Htr 2 Relay Enable Status"], "New Header?"=w1273, "ERD Number"=w1272) -> ("ERD Name Array Out"=w1275:string[], "ERD Number Array Out"=w1274:string[])  [unwired: 13 in]
              n286 = Boolean To (0,1)(Boolean=w1263) -> (0, 1=w1266:i16)
              n287 = Number To Decimal String(number=w1266) -> (decimal integer string=w1254:string)  [unwired: 1 in]
              n288 = Insert Into Array(array=w1269, new element #1=w1260, new element #2=w1259, new element #3=w1258, new element #4=w1257, new element #5=w1256, new element #6=w1255, new element #7=w1254, new element #8=w1253, new element #9=w1252, new element #10=w1251, new element #11=w1250, new element #12=w1249, new element #13=w1248, new element #14=w1247) -> (w1271:string[])  [unwired: 1 in]
            }
            frame 61565 {
              n289 = call "HexStringToBoolean.vi"("Hex String"=w1301) -> ("Boolean"=w1286:bool)
              n290 = call "Build_ERD_Header_String_Array.vi"("ERD Name Array In"=w1295, "ERD Number Array In"=w1294, "ERD Name List"=string[] ["EcoDryInhibitRelay1"], "New Header?"=w1291, "ERD Number"=w1290) -> ("ERD Name Array Out"=w1293:string[], "ERD Number Array Out"=w1292:string[])  [unwired: 13 in]
              n291 = case shown="True" w1286 {
                tunnel: ["False" "True"] -> w1287
                frame False {
                }
                frame True {
                }
              }
              n292 = Insert Into Array(array=w1289, new element=w1287) -> (w1288:string[])  [unwired: 1 in]
              n293 = Bundle By Name(cluster=w1300, "EcoDryInhibitRelay1"=w1286) -> (w1299:T3)
            }
            frame 61566 {
              n294 = call "HexStringToBoolean.vi"("Hex String"=w1324) -> ("Boolean"=w1309:bool)
              n295 = call "Build_ERD_Header_String_Array.vi"("ERD Name Array In"=w1318, "ERD Number Array In"=w1317, "ERD Name List"=string[] ["EcoDryInhibitRelay2"], "New Header?"=w1314, "ERD Number"=w1313) -> ("ERD Name Array Out"=w1316:string[], "ERD Number Array Out"=w1315:string[])  [unwired: 13 in]
              n296 = case shown="True" w1309 {
                tunnel: ["False" "True"] -> w1310
                frame False {
                }
                frame True {
                }
              }
              n297 = Insert Into Array(array=w1312, new element=w1310) -> (w1311:string[])  [unwired: 1 in]
              n298 = Bundle By Name(cluster=w1323, "EcoDryInhibitRelay2"=w1309) -> (w1322:T3)
            }
            frame 61554 {
              n299 = call "HexStringToBoolean.vi"("Hex String"=w1347) -> ("Boolean"=w1332:bool)
              n300 = call "Build_ERD_Header_String_Array.vi"("ERD Name Array In"=w1341, "ERD Number Array In"=w1340, "ERD Name List"=string[] ["OverTempHeaterInhibitRequest"], "New Header?"=w1337, "ERD Number"=w1336) -> ("ERD Name Array Out"=w1339:string[], "ERD Number Array Out"=w1338:string[])  [unwired: 13 in]
              n301 = case shown="True" w1332 {
                tunnel: ["False" "True"] -> w1333
                frame False {
                }
                frame True {
                }
              }
              n302 = Insert Into Array(array=w1335, new element=w1333) -> (w1334:string[])  [unwired: 1 in]
              n303 = Bundle By Name(cluster=w1346, "OverTempHeaterInhibitRequest"=w1332) -> (w1345:T3)
            }
            frame 61555 {
              n304 = call "HexStringToBoolean.vi"("Hex String"=w1370) -> ("Boolean"=w1355:bool)
              n305 = call "Build_ERD_Header_String_Array.vi"("ERD Name Array In"=w1364, "ERD Number Array In"=w1363, "ERD Name List"=string[] ["TrimmerBothCoilInhibitRequest"], "New Header?"=w1360, "ERD Number"=w1359) -> ("ERD Name Array Out"=w1362:string[], "ERD Number Array Out"=w1361:string[])  [unwired: 13 in]
              n306 = case shown="True" w1355 {
                tunnel: ["False" "True"] -> w1356
                frame False {
                }
                frame True {
                }
              }
              n307 = Insert Into Array(array=w1358, new element=w1356) -> (w1357:string[])  [unwired: 1 in]
              n308 = Bundle By Name(cluster=w1369, "TrimBothCoilInhibit"=w1355) -> (w1368:T3)
            }
            frame 61556 {
              n309 = call "HexStringToBoolean.vi"("Hex String"=w1393) -> ("Boolean"=w1378:bool)
              n310 = call "Build_ERD_Header_String_Array.vi"("ERD Name Array In"=w1387, "ERD Number Array In"=w1386, "ERD Name List"=string[] ["NormalHeatControlMethodStatus"], "New Header?"=w1383, "ERD Number"=w1382) -> ("ERD Name Array Out"=w1385:string[], "ERD Number Array Out"=w1384:string[])  [unwired: 13 in]
              n311 = case shown="True" w1378 {
                tunnel: ["False" "True"] -> w1379
                frame False {
                }
                frame True {
                }
              }
              n312 = Insert Into Array(array=w1381, new element=w1379) -> (w1380:string[])  [unwired: 1 in]
              n313 = Bundle By Name(cluster=w1392, "NormalHeatControl"=w1378) -> (w1391:T3)
            }
            frame 61557 {
              n314 = call "HexStringToBoolean.vi"("Hex String"=w1416) -> ("Boolean"=w1401:bool)
              n315 = call "Build_ERD_Header_String_Array.vi"("ERD Name Array In"=w1410, "ERD Number Array In"=w1409, "ERD Name List"=string[] ["FallbackHeatControlMethodStatus"], "New Header?"=w1406, "ERD Number"=w1405) -> ("ERD Name Array Out"=w1408:string[], "ERD Number Array Out"=w1407:string[])  [unwired: 13 in]
              n316 = case shown="True" w1401 {
                tunnel: ["False" "True"] -> w1402
                frame False {
                }
                frame True {
                }
              }
              n317 = Insert Into Array(array=w1404, new element=w1402) -> (w1403:string[])  [unwired: 1 in]
              n318 = Bundle By Name(cluster=w1415, "FallbackHeatControlMethodStatus"=w1401) -> (w1414:T3)
            }
            frame 61567 {
              n319 = call "HexStringToBoolean.vi"("Hex String"=w1439) -> ("Boolean"=w1424:bool)
              n320 = call "Build_ERD_Header_String_Array.vi"("ERD Name Array In"=w1433, "ERD Number Array In"=w1432, "ERD Name List"=string[] ["TrimmerInhibitRelay1"], "New Header?"=w1429, "ERD Number"=w1428) -> ("ERD Name Array Out"=w1431:string[], "ERD Number Array Out"=w1430:string[])  [unwired: 13 in]
              n321 = case shown="True" w1424 {
                tunnel: ["False" "True"] -> w1425
                frame False {
                }
                frame True {
                }
              }
              n322 = Insert Into Array(array=w1427, new element=w1425) -> (w1426:string[])  [unwired: 1 in]
              n323 = Bundle By Name(cluster=w1438, "TrimInhibitR1"=w1424) -> (w1437:T3)
            }
            frame 61568 {
              n324 = call "HexStringToBoolean.vi"("Hex String"=w1462) -> ("Boolean"=w1447:bool)
              n325 = call "Build_ERD_Header_String_Array.vi"("ERD Name Array In"=w1456, "ERD Number Array In"=w1455, "ERD Name List"=string[] ["TrimmerInhibitRelay2"], "New Header?"=w1452, "ERD Number"=w1451) -> ("ERD Name Array Out"=w1454:string[], "ERD Number Array Out"=w1453:string[])  [unwired: 13 in]
              n326 = case shown="True" w1447 {
                tunnel: ["False" "True"] -> w1448
                frame False {
                }
                frame True {
                }
              }
              n327 = Insert Into Array(array=w1450, new element=w1448) -> (w1449:string[])  [unwired: 1 in]
              n328 = Bundle By Name(cluster=w1461, "TrimInhibitR2"=w1447) -> (w1460:T3)
            }
            frame 61582 {
              n329 = call "HexStringToBoolean.vi"("Hex String"=w1485) -> ("Boolean"=w1470:bool)
              n330 = Bundle By Name(cluster=w1484, "Drum Light"=w1470) -> (w1483:T3)
              n331 = case shown="True" w1470 {
                tunnel: ["OFF" "ON"] -> w1480
                frame False {
                }
                frame True {
                }
              }
              n332 = call "Build_ERD_Header_String_Array.vi"("ERD Name Array In"=w1476, "ERD Number Array In"=w1475, "ERD Name List"=string[] ["Drum Light"], "New Header?"=w1472, "ERD Number"=w1471) -> ("ERD Name Array Out"=w1474:string[], "ERD Number Array Out"=w1473:string[])  [unwired: 13 in]
              n333 = Insert Into Array(array=w1479, new element=w1480) -> (w1478:string[])  [unwired: 1 in]
            }
            frame 61594 {
              n334 = Hexadecimal String To Number(string=w1492) -> (number=w1490:u32)  [unwired: 2 in, 1 out]
              n335 = case shown="36" w1490 {
                tunnel: ["Unmapped" ("Motor Profile") "Mixed Load" ("Motor Profile") "Casuals" ("Motor Profile") "Delicates" ("Motor Profile") "Speed Dry" ("Motor Profile") "Jeans" ("Motor Profile") "Timed Dry" ("Motor Profile") "Warm Up" ("Motor Profile") "Air Fluff" ("Motor Profile") "Steam Dewrinkle" ("Motor Profile") "Steam Refresh" ("Motor Profile") "Sanitize Dry" ("Motor Profile") "Bulky Items" ("Motor Profile") "Towels Sheets" ("Motor Profile") "Cottons" ("Motor Profile") "Casuals Less Dry" ("Motor Profile") "Casuals More Dry" ("Motor Profile") "Cottons Less Dry" ("Motor Profile") "Cottons Optimum Dry" ("Motor Profile") "Cottons More Dry" ("Motor Profile") "Delicates Less Dry" ("Motor Profile") "Delicates More Dry" ("Motor Profile") "Time Dry 1" ("Motor Profile") "Time Dry 2" ("Motor Profile") "Time Dry 3" ("Motor Profile") "Time Dry 4" ("Motor Profile") "Time Dry 5" ("Motor Profile") "Time Dry 6" ("Motor Profile") "Active Wear" ("Motor Profile") "DeWrinkle" ("Motor Profile") "EnergySaver" ("Motor Profile") "Washer Link" ("Motor Profile") " BlockedVent" ("Motor Profile") " SmartVent" ("Motor Profile") " Scent" ("Motor Profile") " Max" ("Motor Profile") " Downloaded" ("Motor Profile")] -> w1491
                frame 0, Default {
                }
                frame 1 {
                }
                frame 2 {
                }
                frame 3 {
                }
                frame 4 {
                }
                frame 5 {
                }
                frame 6 {
                }
                frame 7 {
                }
                frame 8 {
                }
                frame 9 {
                }
                frame 10 {
                }
                frame 11 {
                }
                frame 12 {
                }
                frame 13 {
                }
                frame 14 {
                }
                frame 15 {
                }
                frame 16 {
                }
                frame 17 {
                }
                frame 18 {
                }
                frame 19 {
                }
                frame 20 {
                }
                frame 21 {
                }
                frame 22 {
                }
                frame 23 {
                }
                frame 24 {
                }
                frame 25 {
                }
                frame 26 {
                }
                frame 27 {
                }
                frame 28 {
                }
                frame 29 {
                }
                frame 30 {
                }
                frame 31 {
                }
                frame 32 {
                }
                frame 33 {
                }
                frame 34 {
                }
                frame 35 {
                }
                frame 36 {
                }
              }
              n336 = call "Build_ERD_Header_String_Array.vi"("ERD Name Array In"=w1504, "ERD Number Array In"=w1503, "ERD Name List"=w1493, "New Header?"=w1500, "ERD Number"=w1499) -> ("ERD Name Array Out"=w1502:string[], "ERD Number Array Out"=w1501:string[])  [unwired: 13 in]
              n337 = Bundle By Name(cluster=w1508, "Cycle Engine State"=w1491) -> (w1507:T3)
              n338 = Insert Into Array(array=w1498, new element=w1491) -> (w1497:string[])  [unwired: 1 in]
            }
            frame 61597 {
              n339 = Hexadecimal String To Number(string=w1564) -> (number=w1550:u32)  [unwired: 2 in, 1 out]
              n340 = case shown="36" w1550 {
                tunnel: ["Unmapped" ("Motor Profile") "Mixed Load" ("Motor Profile") "Casuals" ("Motor Profile") "Delicates" ("Motor Profile") "Speed Dry" ("Motor Profile") "Jeans" ("Motor Profile") "Timed Dry" ("Motor Profile") "Warm Up" ("Motor Profile") "Air Fluff" ("Motor Profile") "Steam Dewrinkle" ("Motor Profile") "Steam Refresh" ("Motor Profile") "Sanitize Dry" ("Motor Profile") "Bulky Items" ("Motor Profile") "Towels Sheets" ("Motor Profile") "Cottons" ("Motor Profile") "Casuals Less Dry" ("Motor Profile") "Casuals More Dry" ("Motor Profile") "Cottons Less Dry" ("Motor Profile") "Cottons Optimum Dry" ("Motor Profile") "Cottons More Dry" ("Motor Profile") "Delicates Less Dry" ("Motor Profile") "Delicates More Dry" ("Motor Profile") "Time Dry 1" ("Motor Profile") "Time Dry 2" ("Motor Profile") "Time Dry 3" ("Motor Profile") "Time Dry 4" ("Motor Profile") "Time Dry 5" ("Motor Profile") "Time Dry 6" ("Motor Profile") "Active Wear" ("Motor Profile") "DeWrinkle" ("Motor Profile") "EnergySaver" ("Motor Profile") "Washer Link" ("Motor Profile") " BlockedVent" ("Motor Profile") " SmartVent" ("Motor Profile") " Scent" ("Motor Profile") " Max" ("Motor Profile") " Downloaded" ("Motor Profile")] -> w1549
                frame 0, Default {
                }
                frame 1 {
                }
                frame 2 {
                }
                frame 3 {
                }
                frame 4 {
                }
                frame 5 {
                }
                frame 6 {
                }
                frame 7 {
                }
                frame 8 {
                }
                frame 9 {
                }
                frame 10 {
                }
                frame 11 {
                }
                frame 12 {
                }
                frame 13 {
                }
                frame 14 {
                }
                frame 15 {
                }
                frame 16 {
                }
                frame 17 {
                }
                frame 18 {
                }
                frame 19 {
                }
                frame 20 {
                }
                frame 21 {
                }
                frame 22 {
                }
                frame 23 {
                }
                frame 24 {
                }
                frame 25 {
                }
                frame 26 {
                }
                frame 27 {
                }
                frame 28 {
                }
                frame 29 {
                }
                frame 30 {
                }
                frame 31 {
                }
                frame 32 {
                }
                frame 33 {
                }
                frame 34 {
                }
                frame 35 {
                }
                frame 36 {
                }
              }
              n341 = call "Build_ERD_Header_String_Array.vi"("ERD Name Array In"=w1559, "ERD Number Array In"=w1558, "ERD Name List"=w1548, "New Header?"=w1555, "ERD Number"=w1554) -> ("ERD Name Array Out"=w1557:string[], "ERD Number Array Out"=w1556:string[])  [unwired: 13 in]
              n342 = Insert Into Array(array=w1561, new element=w1549) -> (w1560:string[])  [unwired: 1 in]
              n343 = Bundle By Name(cluster=w1565, "Cycle Selected"=w1549) -> (w1566:T3)
            }
            frame 61605 {
              n344 = case shown="\"00\", Default" w1622 {
                tunnel: ["Unknown" "Init" "Selected" "Deselected" "Started" "Stopped" "Paused" "Resumed" "Completed" "Max"] -> w1608
                frame "00", Default {
                }
                frame "01" {
                }
                frame "02" {
                }
                frame "03" {
                }
                frame "04" {
                }
                frame "05" {
                }
                frame "06" {
                }
                frame "07" {
                }
                frame "08" {
                }
                frame "09" {
                }
              }
              n345 = call "Build_ERD_Header_String_Array.vi"("ERD Name Array In"=w1617, "ERD Number Array In"=w1616, "ERD Name List"=string[] ["Sensor Dry Status"], "New Header?"=w1613, "ERD Number"=w1612) -> ("ERD Name Array Out"=w1615:string[], "ERD Number Array Out"=w1614:string[])  [unwired: 13 in]
              n346 = Insert Into Array(array=w1611, new element=w1608) -> (w1610:string[])  [unwired: 1 in]
              n347 = Bundle By Name(cluster=w1623, "Sensor Dry Status"=w1608) -> (w1621:T3)
            }
            frame 61677 {
              n348 = case shown="\"09\"" w1652 {
                tunnel: ["Unknown" "Init" "Selected" "Deselected" "Started" "Paused" "Resumed" "Stopped" "Completed" "Max"] -> w1638
                frame "00", Default {
                }
                frame "01" {
                }
                frame "02" {
                }
                frame "03" {
                }
                frame "04" {
                }
                frame "05" {
                }
                frame "06" {
                }
                frame "07" {
                }
                frame "08" {
                }
                frame "09" {
                }
              }
              n349 = call "Build_ERD_Header_String_Array.vi"("ERD Name Array In"=w1647, "ERD Number Array In"=w1646, "ERD Name List"=string[] ["CoolDownStatus"], "New Header?"=w1643, "ERD Number"=w1642) -> ("ERD Name Array Out"=w1645:string[], "ERD Number Array Out"=w1644:string[])  [unwired: 13 in]
              n350 = Insert Into Array(array=w1641, new element=w1638) -> (w1640:string[])  [unwired: 1 in]
              n351 = Bundle By Name(cluster=w1653, "Cool Down Status"=w1638) -> (w1651:T3)
            }
            frame 61609 {
              n352 = call "HexStringToBoolean.vi"("Hex String"=w1684) -> ("Boolean"=w1669:bool)
              n353 = call "Build_ERD_Header_String_Array.vi"("ERD Name Array In"=w1678, "ERD Number Array In"=w1677, "ERD Name List"=string[] ["TargetMoistureVoltageReached"], "New Header?"=w1674, "ERD Number"=w1673) -> ("ERD Name Array Out"=w1676:string[], "ERD Number Array Out"=w1675:string[])  [unwired: 13 in]
              n354 = case shown="True" w1669 {
                tunnel: ["False" "True"] -> w1670
                frame False {
                }
                frame True {
                }
              }
              n355 = Insert Into Array(array=w1672, new element=w1670) -> (w1671:string[])  [unwired: 1 in]
              n356 = Bundle By Name(cluster=w1683, "Target Voltage Reached"=w1669) -> (w1682:T3)
            }
            frame 61610 {
              n357 = case shown="\"00\", Default" w1704 {
                tunnel: ["N/A" "Empty Drum" "Dry Load" "Cool Down Pasued" "Extended Tumble Paused" "Knob Change" "Power Button Pressed" "Cycle Completed"] -> w1692
                frame "00", Default {
                }
                frame "01" {
                }
                frame "02" {
                }
                frame "03" {
                }
                frame "04" {
                }
                frame "05" {
                }
                frame "06" {
                }
                frame "07" {
                }
              }
              n358 = call "Build_ERD_Header_String_Array.vi"("ERD Name Array In"=w1700, "ERD Number Array In"=w1699, "ERD Name List"=string[] ["EOC Reason"], "New Header?"=w1694, "ERD Number"=w1693) -> ("ERD Name Array Out"=w1698:string[], "ERD Number Array Out"=w1697:string[])  [unwired: 13 in]
              n359 = Insert Into Array(array=w1696, new element=w1692) -> (w1695:string[])  [unwired: 1 in]
              n360 = Bundle By Name(cluster=w1706, "EOC Reason"=w1692) -> (w1705:T3)
            }
            frame 61823 {
              n361 = case shown="\"00\", Default" w1732 {
                tunnel: ["IDLE" "NOT CONNECTED" "COMMISIONING" "COMMISIONING COMPLETE" "RECONNECTING" "CONNECTED"] -> w1721
                frame "00", Default {
                }
                frame "01" {
                }
                frame "02" {
                }
                frame "03" {
                }
                frame "04" {
                }
                frame "05" {
                }
              }
              n362 = call "Build_ERD_Header_String_Array.vi"("ERD Name Array In"=w1729, "ERD Number Array In"=w1728, "ERD Name List"=w1717, "New Header?"=w1723, "ERD Number"=w1722) -> ("ERD Name Array Out"=w1727:string[], "ERD Number Array Out"=w1726:string[])  [unwired: 13 in]
              n363 = Insert Into Array(array=w1725, new element=w1721) -> (w1724:string[])  [unwired: 1 in]
              n364 = Bundle By Name(cluster=w1734, "WiFiCommissioningPSt"=w1721) -> (w1733:T3)
            }
            frame 61615 {
              n365 = case shown="\"00\", Default" w1758 {
                tunnel: ["Unknown" "Small" "Large"] -> w1746
                frame "00", Default {
                }
                frame "01" {
                }
                frame "02" {
                }
              }
              n366 = call "Build_ERD_Header_String_Array.vi"("ERD Name Array In"=w1754, "ERD Number Array In"=w1753, "ERD Name List"=string[] ["LoadSizeByAggregation"], "New Header?"=w1748, "ERD Number"=w1747) -> ("ERD Name Array Out"=w1752:string[], "ERD Number Array Out"=w1751:string[])  [unwired: 13 in]
              n367 = Insert Into Array(array=w1750, new element=w1746) -> (w1749:string[])  [unwired: 1 in]
              n368 = Bundle By Name(cluster=w1760, "Load Size by Ag"=w1746) -> (w1759:T3)
            }
            frame 61613 {
              n369 = case shown="\"00\", Default" w1781 {
                tunnel: ["Unknown" "Small" "Large"] -> w1769
                frame "00", Default {
                }
                frame "01" {
                }
                frame "02" {
                }
              }
              n370 = call "Build_ERD_Header_String_Array.vi"("ERD Name Array In"=w1777, "ERD Number Array In"=w1776, "ERD Name List"=string[] ["Load by Temp"], "New Header?"=w1771, "ERD Number"=w1770) -> ("ERD Name Array Out"=w1775:string[], "ERD Number Array Out"=w1774:string[])  [unwired: 13 in]
              n371 = Insert Into Array(array=w1773, new element=w1769) -> (w1772:string[])  [unwired: 1 in]
              n372 = Bundle By Name(cluster=w1783, "Load Size by Temp"=w1769) -> (w1782:T3)
            }
            frame 61618 {
              n373 = case shown="\"00\", Default" w1804 {
                tunnel: ["Undefined" "Small" "Large"] -> w1792
                frame "00", Default {
                }
                frame "01" {
                }
                frame "02" {
                }
              }
              n374 = call "Build_ERD_Header_String_Array.vi"("ERD Name Array In"=w1800, "ERD Number Array In"=w1799, "ERD Name List"=string[] ["Vent Restriction"], "New Header?"=w1794, "ERD Number"=w1793) -> ("ERD Name Array Out"=w1798:string[], "ERD Number Array Out"=w1797:string[])  [unwired: 13 in]
              n375 = Insert Into Array(array=w1796, new element=w1792) -> (w1795:string[])  [unwired: 1 in]
              n376 = Bundle By Name(cluster=w1806, "Vent Restriction"=w1792) -> (w1805:T3)
            }
            frame 61617 {
              n377 = case shown="\"04\"" w1827 {
                tunnel: ["Idle" "Disabled" "Phase 1Waiting" "Phase 2Waiting" "Phase 3Waiting" "Finished"] -> w1815
                frame "00", Default {
                }
                frame "01" {
                }
                frame "02" {
                }
                frame "03" {
                }
                frame "04" {
                }
                frame "05" {
                }
              }
              n378 = call "Build_ERD_Header_String_Array.vi"("ERD Name Array In"=w1823, "ERD Number Array In"=w1822, "ERD Name List"=string[] ["Dry Load Detection"], "New Header?"=w1817, "ERD Number"=w1816) -> ("ERD Name Array Out"=w1821:string[], "ERD Number Array Out"=w1820:string[])  [unwired: 13 in]
              n379 = Insert Into Array(array=w1819, new element=w1815) -> (w1818:string[])  [unwired: 1 in]
              n380 = Bundle By Name(cluster=w1829, "Dry Load Detection"=w1815) -> (w1828:T3)
            }
            frame 61619 {
              n381 = case shown="\"01\"" w1853 {
                tunnel: ["Disabled" "Idle" "Active" "Complete"] -> w1841
                frame "00", Default {
                }
                frame "01" {
                }
                frame "02" {
                }
                frame "03" {
                }
              }
              n382 = call "Build_ERD_Header_String_Array.vi"("ERD Name Array In"=w1849, "ERD Number Array In"=w1848, "ERD Name List"=string[] ["Restriction Detection Status"], "New Header?"=w1843, "ERD Number"=w1842) -> ("ERD Name Array Out"=w1847:string[], "ERD Number Array Out"=w1846:string[])  [unwired: 13 in]
              n383 = Insert Into Array(array=w1845, new element=w1841) -> (w1844:string[])  [unwired: 1 in]
              n384 = Bundle By Name(cluster=w1855, "Restr Detect Status"=w1841) -> (w1854:T3)
            }
            frame 61624 {
              n385 = call "String Remove All Spaces.vi"("Input String"=w1865) -> ("Spaces Removed"=w1866:string)  [unwired: 13 in, 1 out]
              n386 = Hexadecimal String To Number(string=w1866) -> (number=w1863:u32)  [unwired: 2 in, 1 out]
              n387 = To Unsigned Word Integer(number=w1863) -> (unsigned 16bit integer=w1869:u16)
              n388 = Number To Decimal String(number=w1863) -> (decimal integer string=w1864:string)  [unwired: 1 in]
              n389 = call "Build_ERD_Header_String_Array.vi"("ERD Name Array In"=w1877, "ERD Number Array In"=w1876, "ERD Name List"=string[] ["Raw Moisture"], "New Header?"=w1873, "ERD Number"=w1872) -> ("ERD Name Array Out"=w1875:string[], "ERD Number Array Out"=w1874:string[])  [unwired: 13 in]
              n390 = Insert Into Array(array=w1871, new element=w1864) -> (w1870:string[])  [unwired: 1 in]
              n391 = Bundle By Name(cluster=w1882, "Raw Moisture"=w1869) -> (w1881:T3)
            }
            frame 62214 {
              n392 = call "String Remove All Spaces.vi"("Input String"=w1889) -> ("Spaces Removed"=w1888:string)  [unwired: 13 in, 1 out]
              n393 = Hexadecimal String To Number(string=w1888) -> (number=w1886:u32)  [unwired: 2 in, 1 out]
              n394 = To Unsigned Word Integer(number=w1886) -> (unsigned 16bit integer=w1894:u16)
              n395 = Number To Decimal String(number=w1886) -> (decimal integer string=w1887:string)  [unwired: 1 in]
              n396 = call "Build_ERD_Header_String_Array.vi"("ERD Name Array In"=w1902, "ERD Number Array In"=w1901, "ERD Name List"=string[] ["Raw Inlet ADC"], "New Header?"=w1898, "ERD Number"=w1897) -> ("ERD Name Array Out"=w1900:string[], "ERD Number Array Out"=w1899:string[])  [unwired: 13 in]
              n397 = Insert Into Array(array=w1896, new element=w1887) -> (w1895:string[])  [unwired: 1 in]
              n398 = Bundle By Name(cluster=w1891, "Raw ADC Inlet"=w1894) -> (w1890:T12)
            }
            frame 62215 {
              n399 = call "String Remove All Spaces.vi"("Input String"=w1912) -> ("Spaces Removed"=w1911:string)  [unwired: 13 in, 1 out]
              n400 = Hexadecimal String To Number(string=w1911) -> (number=w1909:u32)  [unwired: 2 in, 1 out]
              n401 = To Unsigned Word Integer(number=w1909) -> (unsigned 16bit integer=w1917:u16)
              n402 = Number To Decimal String(number=w1909) -> (decimal integer string=w1910:string)  [unwired: 1 in]
              n403 = call "Build_ERD_Header_String_Array.vi"("ERD Name Array In"=w1925, "ERD Number Array In"=w1924, "ERD Name List"=string[] ["Raw Outlet ADC"], "New Header?"=w1921, "ERD Number"=w1920) -> ("ERD Name Array Out"=w1923:string[], "ERD Number Array Out"=w1922:string[])  [unwired: 13 in]
              n404 = Insert Into Array(array=w1919, new element=w1910) -> (w1918:string[])  [unwired: 1 in]
              n405 = Bundle By Name(cluster=w1914, "Raw ADC Outlet"=w1917) -> (w1913:T12)
            }
            frame 61626 {
              n406 = case shown="\"08\"" w1947 {
                tunnel: ["Undefined" "Disabled" "Idle" "WaitForFilteredVoltageReset" "Sensing" "Paused" "PausedWhileWaitingForFilteredVoltageReset" "Target Reached" "TargetVoltageReachedByExpiredWatchdog"] -> w1933
                frame "00", Default {
                }
                frame "01" {
                }
                frame "02" {
                }
                frame "03" {
                }
                frame "04" {
                }
                frame "05" {
                }
                frame "06" {
                }
                frame "07" {
                }
                frame "08" {
                }
              }
              n407 = call "Build_ERD_Header_String_Array.vi"("ERD Name Array In"=w1942, "ERD Number Array In"=w1941, "ERD Name List"=string[] ["Check Dampness State"], "New Header?"=w1938, "ERD Number"=w1937) -> ("ERD Name Array Out"=w1940:string[], "ERD Number Array Out"=w1939:string[])  [unwired: 13 in]
              n408 = Insert Into Array(array=w1936, new element=w1933) -> (w1935:string[])  [unwired: 1 in]
              n409 = Bundle By Name(cluster=w1948, "Dampness State"=w1933) -> (w1946:T3)
            }
            frame 61731 {
              n410 = call "HexStringToBoolean.vi"("Hex String"=w1964) -> ("Boolean"=w1963:bool)
              n411 = case shown="True" w1963 {
                tunnel: ["OFF" "ON"] -> w1974
                frame False {
                }
                frame True {
                }
              }
              n412 = call "Build_ERD_Header_String_Array.vi"("ERD Name Array In"=w1970, "ERD Number Array In"=w1969, "ERD Name List"=string[] ["Steam Refresh"], "New Header?"=w1966, "ERD Number"=w1965) -> ("ERD Name Array Out"=w1968:string[], "ERD Number Array Out"=w1967:string[])  [unwired: 13 in]
              n413 = Insert Into Array(array=w1973, new element=w1974) -> (w1972:string[])  [unwired: 1 in]
              n414 = Bundle By Name(cluster=w1978, "Steam Refresh"=w1963) -> (w1977:T3)
            }
            frame 61743 {
              n415 = call "HexStringToBoolean.vi"("Hex String"=w1987) -> ("Boolean"=w1986:bool)
              n416 = case shown="True" w1986 {
                tunnel: ["OFF" "ON"] -> w1997
                frame False {
                }
                frame True {
                }
              }
              n417 = call "Build_ERD_Header_String_Array.vi"("ERD Name Array In"=w1993, "ERD Number Array In"=w1992, "ERD Name List"=string[] ["ReverseDrumInhibitRelay1"], "New Header?"=w1989, "ERD Number"=w1988) -> ("ERD Name Array Out"=w1991:string[], "ERD Number Array Out"=w1990:string[])  [unwired: 13 in]
              n418 = Insert Into Array(array=w1996, new element=w1997) -> (w1995:string[])  [unwired: 1 in]
              n419 = Bundle By Name(cluster=w2001, "ReverseDrumInhibitRelay1"=w1986) -> (w2000:T3)
            }
            frame 61744 {
              n420 = call "HexStringToBoolean.vi"("Hex String"=w2010) -> ("Boolean"=w2009:bool)
              n421 = case shown="True" w2009 {
                tunnel: ["OFF" "ON"] -> w2020
                frame False {
                }
                frame True {
                }
              }
              n422 = call "Build_ERD_Header_String_Array.vi"("ERD Name Array In"=w2016, "ERD Number Array In"=w2015, "ERD Name List"=string[] ["ReverseDrumInhibitRelay2"], "New Header?"=w2012, "ERD Number"=w2011) -> ("ERD Name Array Out"=w2014:string[], "ERD Number Array Out"=w2013:string[])  [unwired: 13 in]
              n423 = Insert Into Array(array=w2019, new element=w2020) -> (w2018:string[])  [unwired: 1 in]
              n424 = Bundle By Name(cluster=w2024, "ReverseDrumInhibitRelay2"=w2009) -> (w2023:T3)
            }
            frame 61956 {
              n425 = Decimal String To Number(string=w2048) -> (number=w2033:i32)  [unwired: 2 in, 1 out]
              n426 = To Unsigned Word Integer(number=w2033) -> (unsigned 16bit integer=w2032:u16)
              n427 = call "Build_ERD_Header_String_Array.vi"("ERD Name Array In"=w2042, "ERD Number Array In"=w2041, "ERD Name List"=string[] ["Raw Moisture"], "New Header?"=w2038, "ERD Number"=w2037) -> ("ERD Name Array Out"=w2040:string[], "ERD Number Array Out"=w2039:string[])  [unwired: 13 in]
              n428 = Number To Decimal String(number=w2033) -> (decimal integer string=w2036:string)  [unwired: 1 in]
              n429 = Insert Into Array(array=w2035, new element=w2036) -> (w2034:string[])  [unwired: 1 in]
              n430 = Bundle By Name(cluster=w2047, "Raw Moisture"=w2032) -> (w2046:T3)
            }
            frame 61719 {
              n431 = call "String Remove All Spaces.vi"("Input String"=w2053) -> ("Spaces Removed"=w2052:string)  [unwired: 13 in, 1 out]
              n432 = Hexadecimal String To Number(string=w2052) -> (number=w2057:u32)  [unwired: 2 in, 1 out]
              n433 = To Unsigned Word Integer(number=w2057) -> (unsigned 16bit integer=w2056:u16)
              n434 = call "Build_ERD_Header_String_Array.vi"("ERD Name Array In"=w2066, "ERD Number Array In"=w2065, "ERD Name List"=string[] ["MaxFilteredMoistureVoltageDuringASensingCycl"], "New Header?"=w2062, "ERD Number"=w2061) -> ("ERD Name Array Out"=w2064:string[], "ERD Number Array Out"=w2063:string[])  [unwired: 13 in]
              n435 = Number To Decimal String(number=w2057) -> (decimal integer string=w2060:string)  [unwired: 1 in]
              n436 = Insert Into Array(array=w2059, new element=w2060) -> (w2058:string[])  [unwired: 1 in]
              n437 = Bundle By Name(cluster=w2071, "MaxFIletered Voltage"=w2056) -> (w2070:T3)
            }
            frame 61968 {
              n438 = call "HexStringToBoolean.vi"("Hex String"=w2092) -> ("Boolean"=w2077:bool)
              n439 = call "Build_ERD_Header_String_Array.vi"("ERD Name Array In"=w2086, "ERD Number Array In"=w2085, "ERD Name List"=string[] ["Centrifugal Switch"], "New Header?"=w2082, "ERD Number"=w2081) -> ("ERD Name Array Out"=w2084:string[], "ERD Number Array Out"=w2083:string[])  [unwired: 13 in]
              n440 = case shown="True" w2077 {
                tunnel: ["OFF" "ON"] -> w2078
                frame False {
                }
                frame True {
                }
              }
              n441 = Insert Into Array(array=w2080, new element=w2078) -> (w2079:string[])  [unwired: 1 in]
              n442 = Bundle By Name(cluster=w2091, "Centrifugal Switch"=w2077) -> (w2090:T3)
            }
            frame 61973 {
              n443 = disable-structure shown="Enabled" {
                disable-tunnel: w2112 -> [w2127 _]
                disable-tunnel: w2111 -> [w2126 w2130]
                disable-tunnel: [w2125 w2130] -> w2110
                disable-tunnel: w2107 -> [w2123 w2129]
                disable-tunnel: w2106 -> [w2122 w2128]
                disable-tunnel: [w2121 w2129] -> w2105
                disable-tunnel: [w2120 w2128] -> w2104
                disable-tunnel: w2103 -> [w2119 _]
                disable-tunnel: w2102 -> [w2118 _]
                disable-tunnel: w2101 -> [w2116 w2131]
                disable-tunnel: [w2115 w2131] -> w2100
                frame Disabled {
                  n444 = Decimal String To Number(string=w2127) -> (number=w2113:i32)  [unwired: 2 in, 1 out]
                  n445 = call "Build_ERD_Header_String_Array.vi"("ERD Name Array In"=w2123, "ERD Number Array In"=w2122, "ERD Name List"=string[] ["Target Dryness"], "New Header?"=w2119, "ERD Number"=w2118) -> ("ERD Name Array Out"=w2121:string[], "ERD Number Array Out"=w2120:string[])  [unwired: 13 in]
                  n446 = To Unsigned Word Integer(number=w2113) -> (unsigned 16bit integer=w2114:u16)
                  n447 = Number To Decimal String(number=w2113) -> (decimal integer string=w2117:string)  [unwired: 1 in]
                  n448 = Insert Into Array(array=w2116, new element=w2117) -> (w2115:string[])  [unwired: 1 in]
                  n449 = Bundle By Name(cluster=w2126, "Target Moisture"=w2114) -> (w2125:T3)
                }
                frame Enabled {
                }
              }
            }
            frame 8193 {
              n450 = Hexadecimal String To Number(string=w2141) -> (number=w2142:u32)  [unwired: 2 in, 1 out]
              n451 = To Unsigned Word Integer(number=w2142) -> (unsigned 16bit integer=w2139:u16)
              n452 = case shown="0, Default" w2139 {
                tunnel: ["NotApplicable" "Drying" "MistSteam" "CoolDown" "ExtendedTumble" "Damp" "AirFluff"] -> w2136
                frame 0, Default {
                }
                frame 128 {
                }
                frame 129 {
                }
                frame 130 {
                }
                frame 131 {
                }
                frame 132 {
                }
                frame 133 {
                }
              }
              n453 = call "Build_ERD_Header_String_Array.vi"("ERD Name Array In"=w2149, "ERD Number Array In"=w2148, "ERD Name List"=w2134, "New Header?"=w2144, "ERD Number"=w2143) -> ("ERD Name Array Out"=w2147:string[], "ERD Number Array Out"=w2146:string[])  [unwired: 13 in]
              n454 = Insert Into Array(array=w2140, new element=w2136) -> (w2135:string[])  [unwired: 1 in]
              n455 = Bundle By Name(cluster=w2138, "Sub-Cycle"=w2136) -> (w2137:T3)
            }
            frame 63489..63508 {
              n456 = call "Build_ERD_Header_String_Array.vi"("ERD Name Array In"=w2175, "ERD Number Array In"=w2174, "ERD Name List"=string[] ["Min Sensing Eapse Time In Sec", "Time Multi Sec X 100", "Time Adder Sec"], "New Header?"=w2171, "ERD Number"=w2170) -> ("ERD Name Array Out"=w2173:string[], "ERD Number Array Out"=w2172:string[])  [unwired: 13 in]
              n457 = call "Parse Any Restric Data.vi"("Data"=w2167, "ERD_Always Show in"=w2169) -> ("CSV Data Out"=w2164:string[], "ERD_Always Show out"=w2168:T3)  [unwired: 7 in, 1 out]
              n458 = Insert Into Array(array=w2166, new element=w2164) -> (w2165:string[])  [unwired: 1 in]
            }
            frame 59 {
              n459 = call "VersionConversionData.vi"("Version In"=w2182) -> ("Version Out"=w2181:string)  [unwired: 9 in, 1 out]
              n460 = call "Build_ERD_Header_String_Array.vi"("ERD Name Array In"=w2193, "ERD Number Array In"=w2192, "ERD Name List"=string[] ["ParametricVersion"], "New Header?"=w2189, "ERD Number"=w2188) -> ("ERD Name Array Out"=w2191:string[], "ERD Number Array Out"=w2190:string[])  [unwired: 13 in]
              n461 = Bundle By Name(cluster=w2200, "Parametric Version"=w2181) -> (w2199:T2)
              n462 = Insert Into Array(array=w2196, new element=w2181) -> (w2195:string[])  [unwired: 1 in]
            }
            frame 8397 {
              n463 = case shown="\"99\", Default" w2205 {
                selector: w2205 -> [_ _ w2225 _]
                tunnel: ["LOCKED" ("Write Access") "REQUESTED" ("Write Access") w2224 "UNLOCKED" ("Write Access")] -> w2201
                frame "01" {
                }
                frame "FF" {
                }
                frame "99", Default {
                  n464 = Concatenate Strings(w2225, "-UNKNOWN" ("Write Access")) -> (w2224:string)
                }
                frame "00" {
                }
              }
              n465 = Build Array("WriteAccessRequest" ("String")) -> (w2206:string[])
              n466 = call "Build_ERD_Header_String_Array.vi"("ERD Name Array In"=w2217, "ERD Number Array In"=w2216, "ERD Name List"=w2206, "New Header?"=w2213, "ERD Number"=w2212) -> ("ERD Name Array Out"=w2215:string[], "ERD Number Array Out"=w2214:string[])  [unwired: 13 in]
              n467 = Bundle By Name(cluster=w2203, "Write Access Request"=w2201) -> (w2202:T10)
              n468 = Insert Into Array(array=w2219, new element=w2201) -> (w2218:string[])  [unwired: 1 in]
            }
            frame 8398 {
              n469 = case shown="\"99\", Default" w2233 {
                selector: w2233 -> [_ _ w2253 _]
                tunnel: ["LOCKED" ("Write Access") "REQUESTED" ("Write Access") w2251 "UNLOCKED" ("Write Access")] -> w2228
                frame "01" {
                }
                frame "FF" {
                }
                frame "99", Default {
                  n470 = Concatenate Strings(w2253, "-UNKNOWN" ("Write Access")) -> (w2251:string)
                }
                frame "00" {
                }
              }
              n471 = Build Array("RJ45WriteAccessActual" ("String")) -> (w2234:string[])
              n472 = call "Build_ERD_Header_String_Array.vi"("ERD Name Array In"=w2244, "ERD Number Array In"=w2243, "ERD Name List"=w2234, "New Header?"=w2240, "ERD Number"=w2239) -> ("ERD Name Array Out"=w2242:string[], "ERD Number Array Out"=w2241:string[])  [unwired: 13 in]
              n473 = Bundle By Name(cluster=w2231, "Write Access Actual"=w2228) -> (w2230:T10)
              n474 = Insert Into Array(array=w2246, new element=w2228) -> (w2245:string[])  [unwired: 1 in]
            }
            frame 65522 {
              n475 = case shown="\"00\"" w2260 {
                selector: w2260 -> [_ w2279 _]
                tunnel: ["LOCKED" ("Write Access") w2277 "UNLOCKED" ("Write Access")] -> w2255
                frame "01" {
                }
                frame "99", Default {
                  n476 = Concatenate Strings(w2279, "-UNKNOWN" ("Write Access")) -> (w2277:string)
                }
                frame "00" {
                }
              }
              n477 = Build Array("Rj45LockedAtLeastOnce" ("String")) -> (w2261:string[])
              n478 = call "Build_ERD_Header_String_Array.vi"("ERD Name Array In"=w2271, "ERD Number Array In"=w2270, "ERD Name List"=w2261, "New Header?"=w2267, "ERD Number"=w2266) -> ("ERD Name Array Out"=w2269:string[], "ERD Number Array Out"=w2268:string[])  [unwired: 13 in]
              n479 = Bundle By Name(cluster=w2258, "LockedAtLeastOnce"=w2255) -> (w2257:T10)
              n480 = Insert Into Array(array=w2273, new element=w2255) -> (w2272:string[])  [unwired: 1 in]
            }
            frame 8351 {
              n481 = String Subset(string=w2282, offset (0)=0, length (rest)=12 ("length (rest)")) -> (substring=w2287:string)
              n482 = String Subset(string=w2282, offset (0)=12, length (rest)=2 ("length (rest)")) -> (substring=w2293:string)
              n483 = String Subset(string=w2282, offset (0)=15, length (rest)=2 ("length (rest)")) -> (substring=w2296:string)
              n484 = String Subset(string=w2282, offset (0)=18, length (rest)=2 ("length (rest)")) -> (substring=w2299:string)
              n485 = String Subset(string=w2282, offset (0)=21, length (rest)=2 ("length (rest)")) -> (substring=w2302:string)
              n486 = String Subset(string=w2282, offset (0)=84, length (rest)=2 ("length (rest)")) -> (substring=w2288:string)
              n487 = case shown="\"0B\"" w2293 {
                selector: w2293 -> [_ _ _ _ _ _ _ _ _ _ _ _ w2373]
                tunnel: ["IDLE" ("Write Access") "RESERVED" ("Write Access") "CYCLE REQUEST" ("Write Access") "CYCLE STARTED" ("Write Access") "PAUSED" ("Write Access") "SESSION EXPIRED" ("Write Access") "Authorized" ("Write Access") "DENIED" ("Write Access") "FAULT" ("Write Access") "SESSION CANCELLED" ("Write Access") "CYCLE COMPLETE" ("Write Access") "COINBOX" ("Write Access") w2371] -> w2286
                frame "00" {
                }
                frame "01" {
                }
                frame "02" {
                }
                frame "03" {
                }
                frame "04" {
                }
                frame "05" {
                }
                frame "06" {
                }
                frame "07" {
                }
                frame "08" {
                }
                frame "09" {
                }
                frame "0A" {
                }
                frame "0B" {
                }
                frame "FF", Default {
                  n488 = Concatenate Strings(w2373, " -UnKnown" ("Write Access")) -> (w2371:string)
                }
              }
              n489 = case shown="\"07\"" w2296 {
                selector: w2296 -> [w2348 _ _ _ _ _ _ _ _ _ _]
                tunnel: [w2346 "WaterHeater" ("Write Access") "ClothesDryer" ("Write Access") "ClothesWasher" ("Write Access") "Refrigerator" ("Write Access") "Microwave" ("Write Access") "Advantium" ("Write Access") "Dishwasher" ("Write Access") "Oven" ("Write Access") "ElectricRange" ("Write Access") "Gas Range" ("Write Access")] -> w2285
                frame "FF", Default {
                  n490 = Concatenate Strings(w2348, " -UnKnown" ("Write Access")) -> (w2346:string)
                }
                frame "00" {
                }
                frame "01" {
                }
                frame "02" {
                }
                frame "03" {
                }
                frame "04" {
                }
                frame "05" {
                }
                frame "06" {
                }
                frame "07" {
                }
                frame "08" {
                }
                frame "09" {
                }
              }
              n491 = case shown="\"09\"" w2299 {
                selector: w2299 -> [w2332 _ _ _ _ _ _ _ _ _ _ _ _ _]
                tunnel: [w2330 "NotDefined" ("Write Access") "BasketClean" ("Write Access") "DrainSpin" ("Write Access") "QuickRinse" ("Write Access") "BulkyItems" ("Write Access") "Sanitize" ("Write Access") "TowelsSheets" ("Write Access") "WasherSteamRefresh" ("Write Access") "NormalMixedLoad" ("Write Access") "Whites" ("Write Access") "DarkColors" ("Write Access") "Jeans" ("Write Access") "HandWash" ("Write Access")] -> w2284
                frame "FF", Default {
                  n492 = Concatenate Strings(w2332, " -UnKnown" ("Write Access")) -> (w2330:string)
                }
                frame "00" {
                }
                frame "01" {
                }
                frame "02" {
                }
                frame "03" {
                }
                frame "04" {
                }
                frame "05" {
                }
                frame "06" {
                }
                frame "07" {
                }
                frame "08" {
                }
                frame "09" {
                }
                frame "10" {
                }
                frame "11" {
                }
                frame "12" {
                }
              }
              n493 = case shown="\"FF\", Default" w2302 {
                selector: w2302 -> [w2325 _ _ _ _]
                tunnel: [w2323 "UnKnown" ("Write Access") "TopLoad" ("Write Access") "FrontLoad" ("Write Access") "TopLoad S2" ("Write Access")] -> w2283
                frame "FF", Default {
                  n494 = Concatenate Strings(w2325, " -UnKnown" ("Write Access")) -> (w2323:string)
                }
                frame "00" {
                }
                frame "01" {
                }
                frame "02" {
                }
                frame "03" {
                }
              }
              n495 = Build Array("CommercialLaundryStatus" ("String")) -> (w2309:string[])
              n496 = call "Build_ERD_Header_String_Array.vi"("ERD Name Array In"=w2318, "ERD Number Array In"=w2317, "ERD Name List"=w2309, "New Header?"=w2314, "ERD Number"=w2313) -> ("ERD Name Array Out"=w2316:string[], "ERD Number Array Out"=w2315:string[])  [unwired: 13 in]
              n497 = Bundle By Name(cluster=w2305, "Session"=w2287, "Phase"=w2286, "Appliance Type"=w2285, "Cycle Selected"=w2284, "Platform Type"=w2283, "Retry Signal"=w2288) -> (w2281:T8)
              n498 = Insert Into Array(array=w2320, new element=w2282) -> (w2319:string[])  [unwired: 1 in]
            }
            frame 8350 {
              # "CycleComplete"
              n499 = String Subset(string=w2375, offset (0)=0, length (rest)=12 ("length (rest)")) -> (substring=w2380:string)
              n500 = String Subset(string=w2375, offset (0)=12, length (rest)=2 ("length (rest)")) -> (substring=w2386:string)
              n501 = String Subset(string=w2375, offset (0)=15, length (rest)=2 ("length (rest)")) -> (substring=w2389:string)
              n502 = String Subset(string=w2375, offset (0)=18, length (rest)=2 ("length (rest)")) -> (substring=w2392:string)
              n503 = String Subset(string=w2375, offset (0)=21, length (rest)=2 ("length (rest)")) -> (substring=w2395:string)
              n504 = String Subset(string=w2375, offset (0)=84, length (rest)=2 ("length (rest)")) -> (substring=w2381:string)
              n505 = case shown="\"0B\"" w2386 {
                selector: w2386 -> [_ _ _ _ _ _ _ _ _ _ _ w2464 _]
                tunnel: ["RESERVED" ("Write Access") "CYCLE REQUEST" ("Write Access") "CYCLE STARTED" ("Write Access") "PAUSED" ("Write Access") "SESSION EXPIRED" ("Write Access") "Authorized" ("Write Access") "DENIED" ("Write Access") "FAULT" ("Write Access") "SESSION CANCELLED" ("Write Access") "CYCLE COMPLETE" ("Write Access") "COINBOX" ("Write Access") w2462 "IDLE" ("Write Access")] -> w2379
                frame "01" {
                }
                frame "02" {
                }
                frame "03" {
                }
                frame "04" {
                }
                frame "05" {
                }
                frame "06" {
                }
                frame "07" {
                }
                frame "08" {
                }
                frame "09" {
                }
                frame "0A" {
                }
                frame "0B" {
                }
                frame "FF", Default {
                  n506 = Concatenate Strings(w2464, " -UnKnown" ("Write Access")) -> (w2462:string)
                }
                frame "00" {
                }
              }
              n507 = case shown="\"FF\", Default" w2389 {
                selector: w2389 -> [w2440 _ _ _ _ _ _ _ _ _ _]
                tunnel: [w2438 "WaterHeater" ("Write Access") "ClothesDryer" ("Write Access") "ClothesWasher" ("Write Access") "Refrigerator" ("Write Access") "Microwave" ("Write Access") "Advantium" ("Write Access") "Dishwasher" ("Write Access") "Oven" ("Write Access") "ElectricRange" ("Write Access") "Gas Range" ("Write Access")] -> w2378
                frame "FF", Default {
                  n508 = Concatenate Strings(w2440, " -UnKnown" ("Write Access")) -> (w2438:string)
                }
                frame "00" {
                }
                frame "01" {
                }
                frame "02" {
                }
                frame "03" {
                }
                frame "04" {
                }
                frame "05" {
                }
                frame "06" {
                }
                frame "07" {
                }
                frame "08" {
                }
                frame "09" {
                }
              }
              n509 = case shown="\"FF\", Default" w2392 {
                selector: w2392 -> [w2424 _ _ _ _ _ _ _ _ _ _ _ _ _]
                tunnel: [w2422 "NotDefined" ("Write Access") "BasketClean" ("Write Access") "DrainSpin" ("Write Access") "QuickRinse" ("Write Access") "BulkyItems" ("Write Access") "Sanitize" ("Write Access") "TowelsSheets" ("Write Access") "WasherSteamRefresh" ("Write Access") "NormalMixedLoad" ("Write Access") "Whites" ("Write Access") "DarkColors" ("Write Access") "Jeans" ("Write Access") "HandWash" ("Write Access")] -> w2377
                frame "FF", Default {
                  n510 = Concatenate Strings(w2424, " -UnKnown" ("Write Access")) -> (w2422:string)
                }
                frame "00" {
                }
                frame "01" {
                }
                frame "02" {
                }
                frame "03" {
                }
                frame "04" {
                }
                frame "05" {
                }
                frame "06" {
                }
                frame "07" {
                }
                frame "08" {
                }
                frame "09" {
                }
                frame "10" {
                }
                frame "11" {
                }
                frame "12" {
                }
              }
              n511 = case shown="\"FF\", Default" w2395 {
                selector: w2395 -> [w2418 _ _ _]
                tunnel: [w2416 "UnKnown" ("Write Access") "TopLoad" ("Write Access") "FrontLoad" ("Write Access")] -> w2376
                frame "FF", Default {
                  n512 = Concatenate Strings(w2418, " -UnKnown" ("Write Access")) -> (w2416:string)
                }
                frame "00" {
                }
                frame "01" {
                }
                frame "02" {
                }
              }
              n513 = Build Array("CommercialLaundryStatusExternal" ("String")) -> (w2402:string[])
              n514 = call "Build_ERD_Header_String_Array.vi"("ERD Name Array In"=w2411, "ERD Number Array In"=w2410, "ERD Name List"=w2402, "New Header?"=w2407, "ERD Number"=w2406) -> ("ERD Name Array Out"=w2409:string[], "ERD Number Array Out"=w2408:string[])  [unwired: 13 in]
              n515 = Bundle By Name(cluster=w2398, "Session Ext"=w2380, "Phase Ext"=w2379, "Appliance Type Ext"=w2378, "Cycle Selected Ext"=w2377, "Platform Type Ext"=w2376, "Retry Signal Ext"=w2381) -> (w2374:T8)
              n516 = Insert Into Array(array=w2413, new element=w2375) -> (w2412:string[])  [unwired: 1 in]
            }
            frame 61976 {
              n517 = case shown="\"02\"" w2469 {
                tunnel: ["APP" "Coin" "NotDefined"] -> w2466
                frame "01" {
                }
                frame "02" {
                }
                frame "00", Default {
                }
              }
              n518 = call "Build_ERD_Header_String_Array.vi"("ERD Name Array In"=w2475, "ERD Number Array In"=w2474, "ERD Name List"=w2473, "New Header?"=w2479, "ERD Number"=w2478) -> ("ERD Name Array Out"=w2477:string[], "ERD Number Array Out"=w2476:string[])  [unwired: 13 in]
              n519 = Bundle By Name(cluster=w2471, "Payment Method"=w2466) -> (w2470:T3)
              n520 = Insert Into Array(array=w2468, new element=w2466) -> (w2467:string[])  [unwired: 1 in]
            }
          }
          "Numeric" <- w53
        }
        n521 = in-place-cluster #1("CSV File String Arrays.ERD Name Array"=w29, "CSV File String Arrays.ERD Number Array"=w28, "Version"=w38, "ERD_Always Show"=w37, "Personality Set"=w35, "CSV File String Arrays.ERD Converted String Data"=w30, "Heat Control"=w27, "Temp ADC"=w26, "Boot Loader Version"=w23, "RJ45"=w20, "Commercial_Laundry"=w18) -> (w10:T1)
      }
    }
    frame Error {
      n522 = Unbundle By Name(w2491) -> ("code"=w2495:i32, "status"=w2496:bool, "source"=w2493:string)
      n523 = Equal?(x=w2495, y=-5006) -> (x = y?=w2499:bool)
      n524 = case shown="True" w2499 {
        tunnel: [w2503 FALSE] -> w2497
        tunnel: w2496 -> [w2503 _]
        tunnel: w2495 -> [w2502 w2505]
        tunnel: [w2502 w2505] -> w2494
        tunnel: [w2501 w2504] -> w2492
        tunnel: w2493 -> [w2501 w2504]
        frame False {
        }
        frame True {
        }
      }
      n525 = Bundle By Name(cluster=errorcluster {"status"=FALSE, "code"=0, "source"=""} ("error constant"), "status"=w2497, "code"=w2494, "source"=w2492) -> (w2490:errorcluster)
    }
  }
  "Error Out" <- w5
  "All_ERD_Data_Bundled_Brass" <- w4
